vi "Build Do.vi"(4 "BuildType":T1 items=["simple", "Dialog", "PVUpdate", "Dialog&PV", "Asynch", "AsynchDial", "Ack"], 6 "Wiring Spec":T2, 8 "error in (no error)":errorcluster, 10 "Do VI":refnum<vi>, 11 "CS++Actor in":refnum<class "CS++Actor.lvclass">) -> (0 "error out":errorcluster, 3 "CS++Actor out":refnum<class "CS++Actor.lvclass">)   [LabVIEW 2016, in "CS++Actor.lvlib" / "CS++Actor.lvclass"]
doc: "Creates the Do.vi for the new message."
uses:
  CS++Actor.lvclass
  CSPP_MessageMakerMain/BuildType.ctl
  CS++Actor.lvclass/CS++Actor.ctl
  <vilib>/Utility/traverseref.llb/TRef TravTarget.ctl
  <vilib>/Utility/miscctls.llb/LVPositionTypeDef.ctl
  <vilib>/Utility/Data Type/Type Definitions/Data Type.ctl
  <vilib>/Utility/traverseref.llb/VI Scripting - Traverse.lvlib
  <vilib>/Utility/Data Type/NI_Data Type.lvlib
  CSPP_MessageMakerMain/CS++MessageMakerMain.lvclass
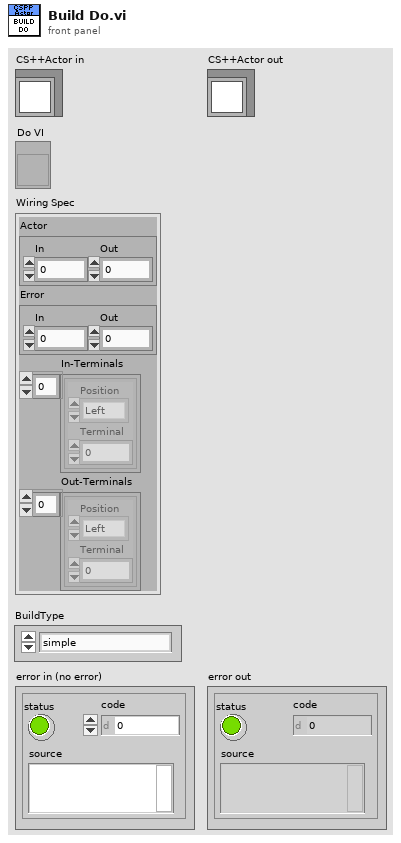
[diagram p1: front panel]
types:
  T1 = typedef "CS++MessageMakerMain.lvlib/CS++MessageMakerMain.lvclass/BuildType.ctl" = u16
  T2 = cluster{"Actor":cluster{"In":i32, "Out":i32}, "Error":cluster{"In":i32, "Out":i32}, "In-Terminals":cluster{"Position":enum16{"Left", "Top", "Bottom", "Right"}, "Terminal":i32}[], "Out-Terminals":cluster{"Position":enum16{"Left", "Top", "Bottom", "Right"}, "Terminal":i32}[]}
  T3 = enum16{"Replace Class Controls/Constants", "Prepare SubVI", "Wire Method Inputs", "Replace Msg Ctrl if necessary", "Create DynamicDispatch Control", "Create PseudoTypedef", "Connect Pre (Un)Bundler", "Replace PV VIs", "RedoWiring", "Connect MethodOut to Bundler", "Delete AsynchAndNoPara", "DeleteBoolDIMConversion"}
  T4 = typedef "TRef TravTarget.ctl" = enum16{"FP", "BD", "Other"}
  T5 = enum16{"Invalid Wire Rule", "Required", "Recommended", "Optional", "Dynamic Dispatch"}
  T6 = typedef "LVPositionTypeDef.ctl" = cluster{"Left":i32, "Top":i32}
  T7 = typedef "NI_Data Type.lvlib/Data Type.ctl" = enum8{"Invalid Type", "Void", "I8", "I16", "I32", "I64", "U8", "U16", "U32", "U64", "Single Float", "Double Float", "Extended Float", "Single Complex", "Double Complex", "Extended Complex", "Enum U8", "Enum U16", "Enum U32", "Enum U64", "Single Float With Unit", "Double Float With Unit", "Extended Float With Unit", "Single Complex with Unit", "Double Complex with Unit", "Extended Complex with Unit", "Boolean", "String", "Path", "Picture", "Tag", "Array", "Cluster", "Variant", "LV Variant", "Waveform", "Timestamp", "Digital Waveform", "Digital Data", "ExpressData", "Refnum", "External Data", "VI", "Poly VI", "LabVIEW Class Instance", "Fixed Point"}
  T8 = cluster{"Position":enum16{"Left", "Top", "Bottom", "Right"}, "Terminal":i32}[]
  T9 = cluster{"Position":enum16{"Left", "Top", "Bottom", "Right"}, "Terminal":i32}
  T10 = enum16{"Invalid Wire Rule", "Required", "Recommended", "Optional", "Dynamic Dispatch"}[]
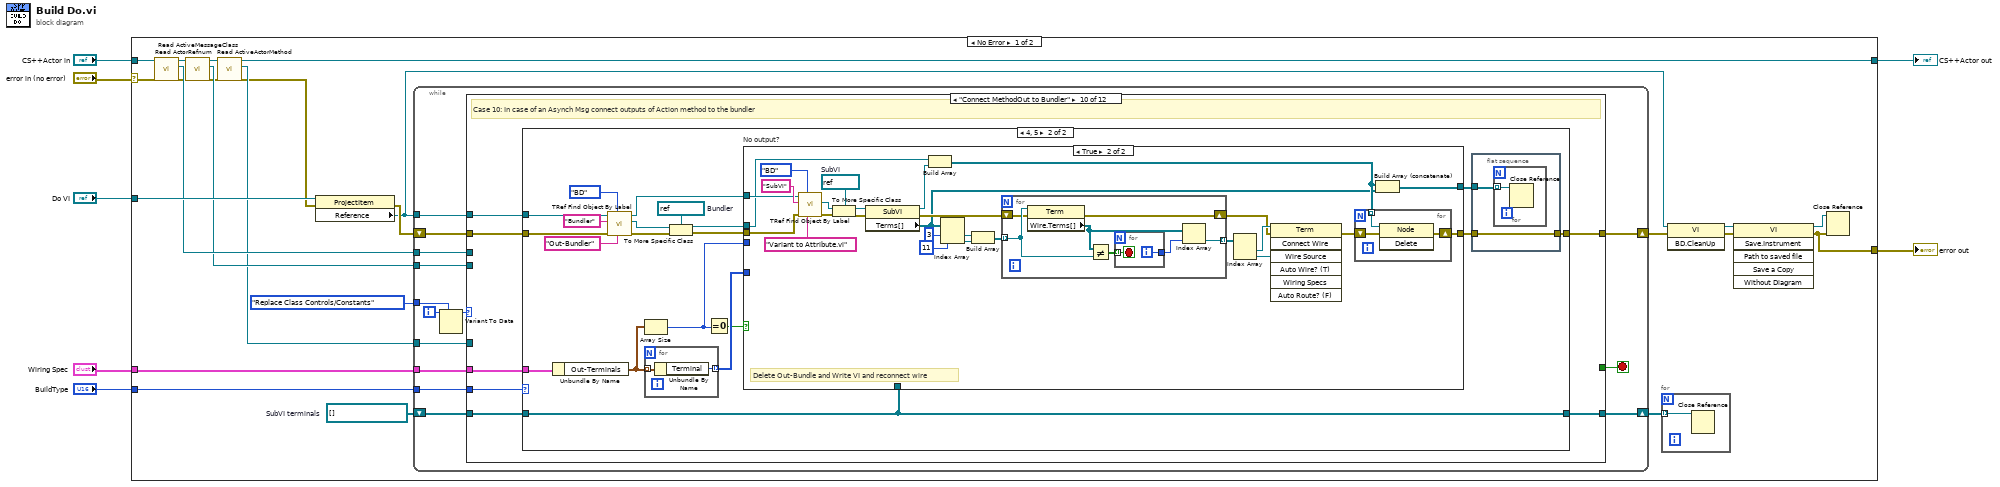
[diagram p0: block diagram]
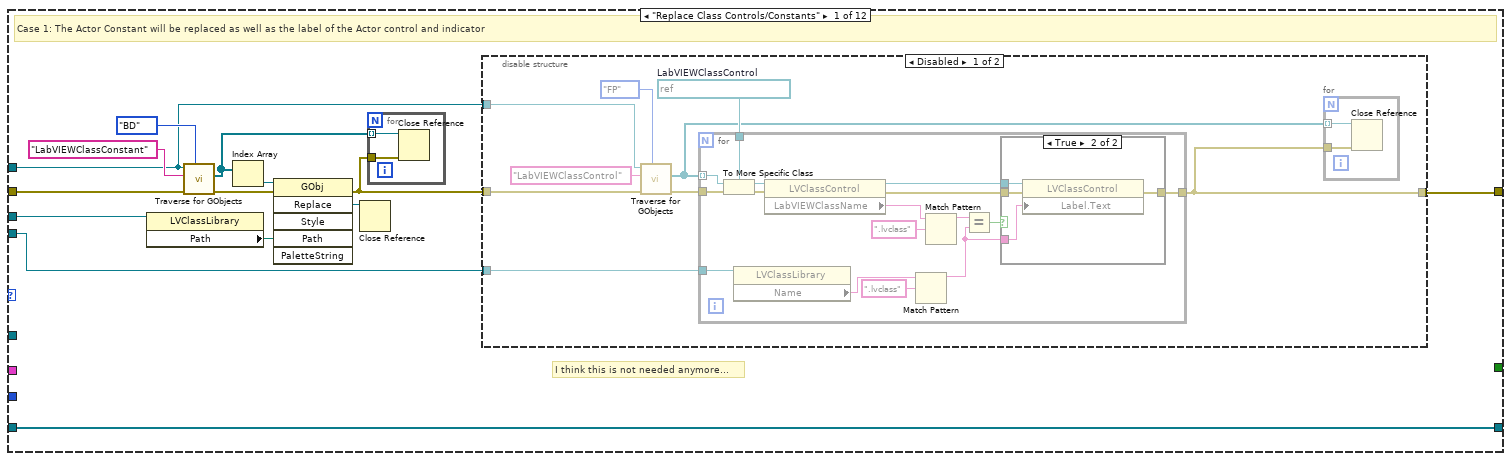
[diagram p2: hidden frame]
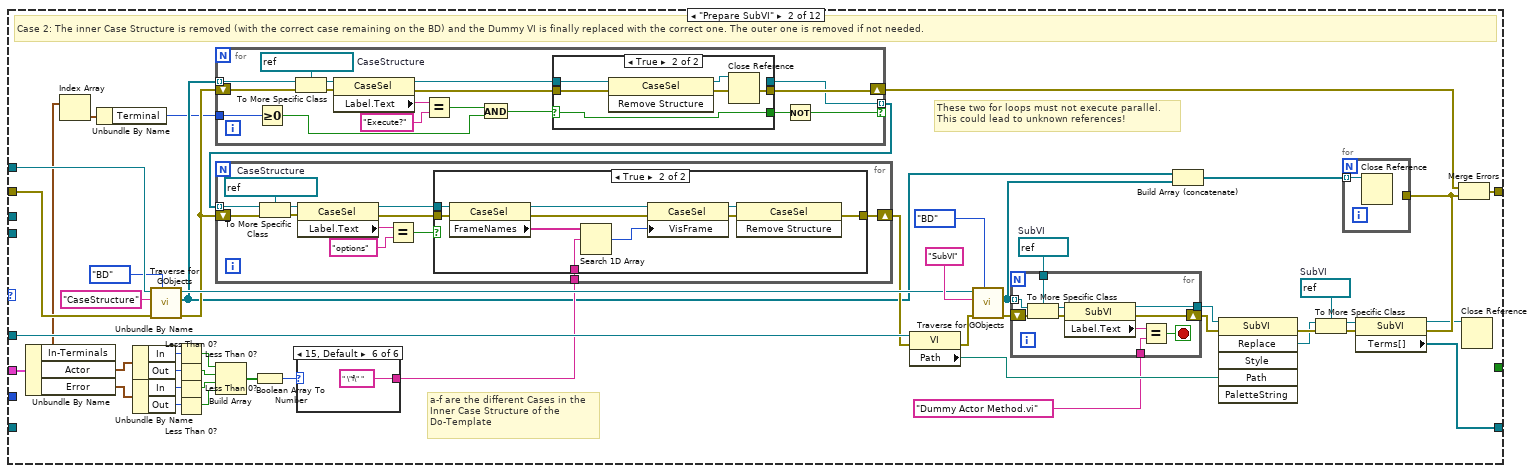
[diagram p5: hidden frame]
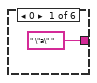
[diagram p8: hidden frame]
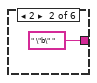
[diagram p9: hidden frame]
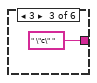
[diagram p10: hidden frame]
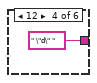
[diagram p11: hidden frame]
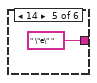
[diagram p12: hidden frame]
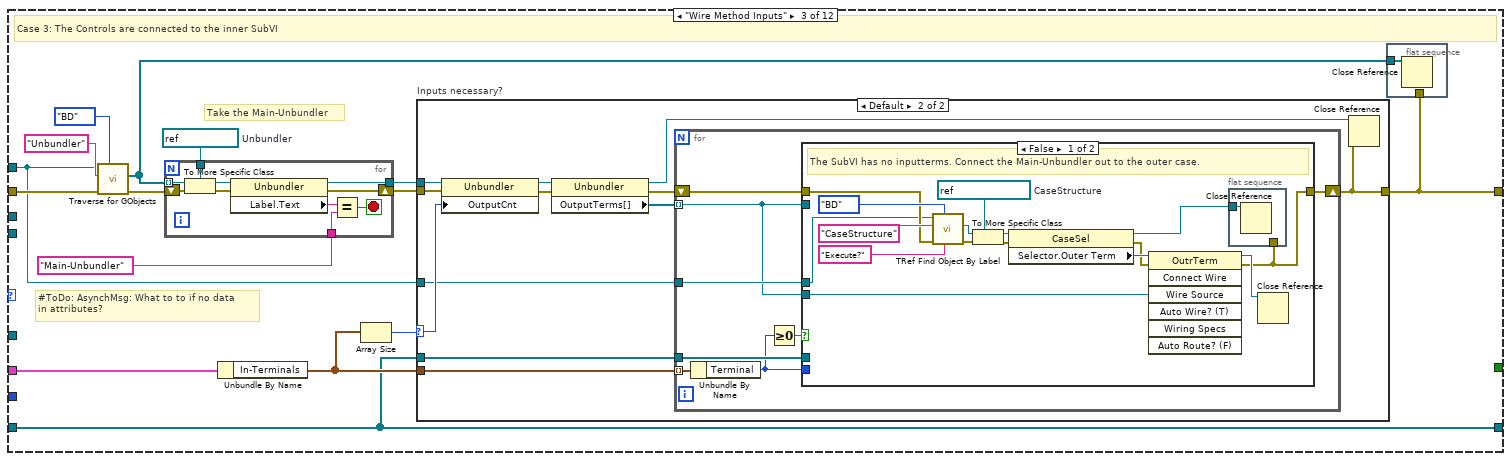
[diagram p13: hidden frame]
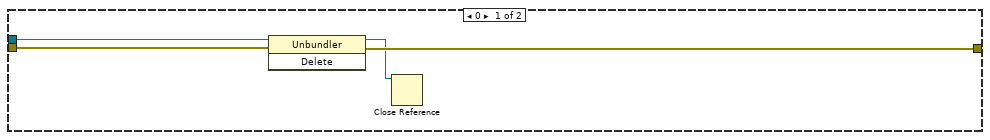
[diagram p14: hidden frame]
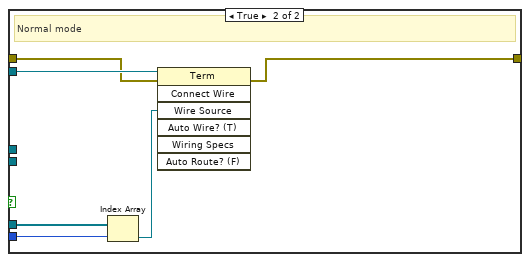
[diagram p15: hidden frame]
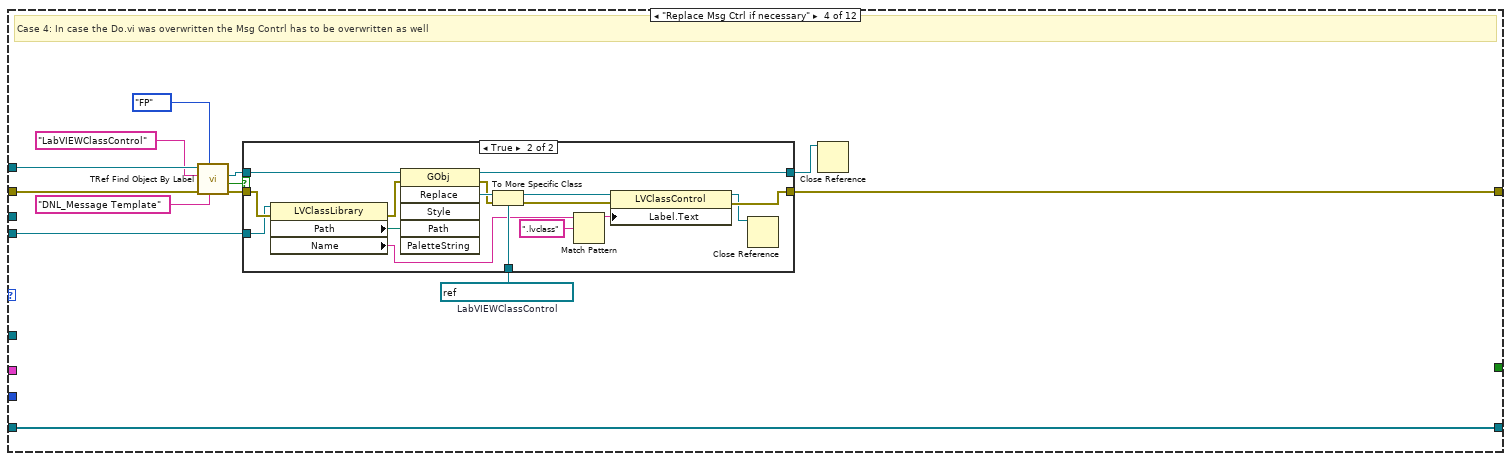
[diagram p16: hidden frame]
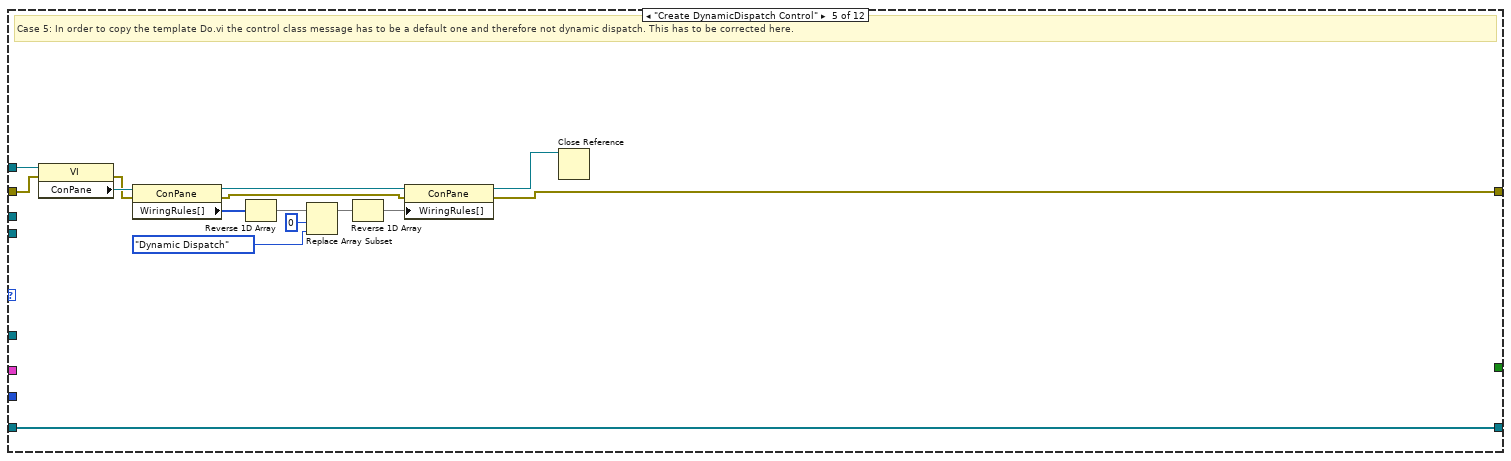
[diagram p18: hidden frame]
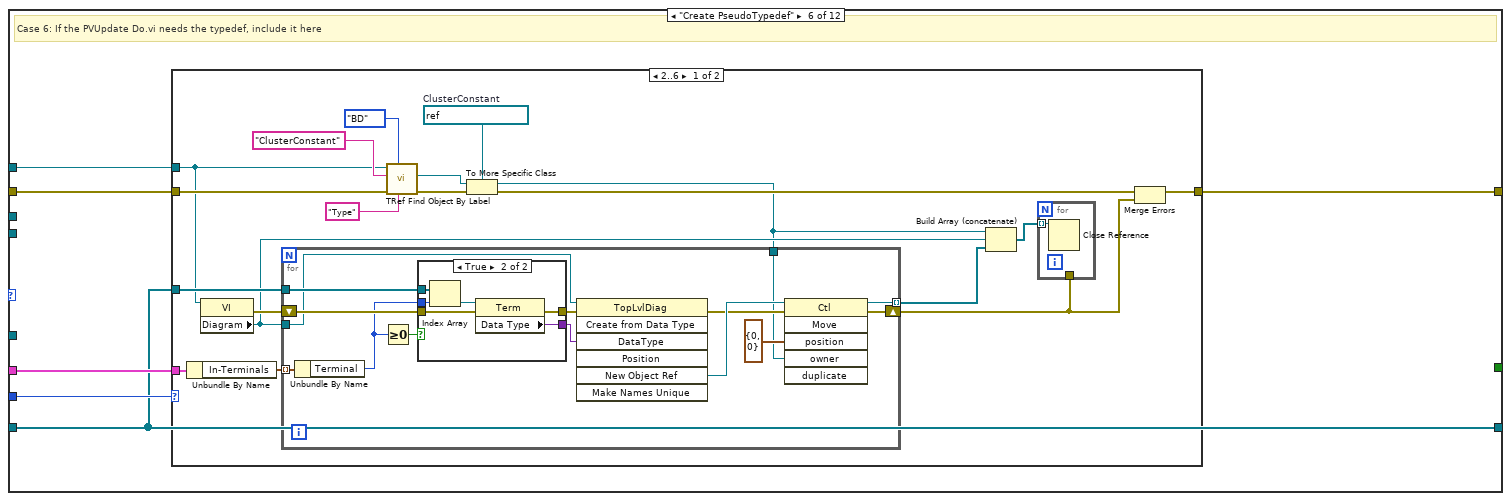
[diagram p19: hidden frame]
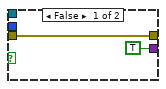
[diagram p20: hidden frame]
diagram:
  n1 = case shown="No Error" "error in (no error)" {
    selector: "error in (no error)" -> [w14 w1120]
    tunnel: "Do VI" -> [w31 _]
    tunnel: "Wiring Spec" -> [w29 _]
    tunnel: [w10 w1120] -> w5
    tunnel: "CS++Actor in" -> [w24 w1121]
    tunnel: [w15 w1121] -> w3
    tunnel: "BuildType" -> [w9 _]
    frame No Error {
      w8 = refnum<vi>[] []  # SubVI terminals
      n2 = call "Read ActorRefnum.vi"("error in (no error)"=w14, "CS++Actor in"=w24) -> ("error out"=w21:errorcluster, "ActorRefnum"=w23:refnum<vi>, "CS++Actor out"=w22:refnum<class "CS++Actor.lvclass">)  [unwired: 7 in]
      n3 = call "Read ActiveMessageClass.vi"("error in (no error)"=w21, "CS++Actor in"=w22) -> ("error out"=w18:errorcluster, "ActiveMessageClass"=w20:refnum<vi>, "CS++Actor out"=w19:refnum<class "CS++Actor.lvclass">)  [unwired: 7 in]
      n4 = call "Read ActiveActorMethod.vi"("error in (no error)"=w18, "CS++Actor in"=w19) -> ("error out"=w16:errorcluster, "ActiveActorMethod"=w17:refnum<vi>, "CS++Actor out"=w15:refnum<class "CS++Actor.lvclass">)  [unwired: 7 in]
      n5 = property class="ProjectItem"(reference=w31, error in=w16) -> (error out=w30:errorcluster, "Reference"=w25:refnum<vi>)  [unwired: 1 out]
      n6 = while {
        tunnel: w25 -> [w46]
        tunnel: w29 -> [w44]
        shift-right: [w43] -> w28
        shift-left: w30 -> [w45]
        tunnel: T3."Replace Class Controls/Constants" -> [w41]
        tunnel: w23 -> [w39]
        tunnel: w17 -> [w38]
        shift-right: [w36] -> w26
        shift-left: w8 -> [w35]
        tunnel: w20 -> [w34]
        tunnel: w9 -> [w33]
        i -> [w42]
        stop <- w37 stop-if-true
        n7 = Variant To Data(type=w41, Variant=w42) -> (data=w40:T3)  [unwired: 1 in, 1 out]
        n8 = case shown="\"Connect MethodOut to Bundler\"" w40 {
          tunnel: w46 -> [w49 w143 w210 w292 w325 w330 w380 w440 w588 w739 w854 w937]
          tunnel: w45 -> [w54 w142 w218 w293 w326 w333 w379 w438 w589 w738 w855 w938]
          tunnel: w44 -> [_ w141 w221 _ _ w329 _ _ _ w737 w853 _]
          tunnel: [w47 w101 w212 w285 w313 w332 w378 w439 w590 w736 w856 w939] -> w43
          tunnel: w39 -> [w55 _ _ _ _ _ _ w437 _ _ _ _]
          tunnel: w38 -> [_ w140 _ _ _ _ _ _ _ _ _ _]
          tunnel: [_ _ _ _ _ _ _ _ _ _ _ TRUE] -> w37
          tunnel: [w51 w139 w209 w294 w327 w328 w381 w441 w592 w742 w858 w941] -> w36
          tunnel: w35 -> [w51 _ w209 w294 w327 w328 w381 w441 w592 w741 w858 w941]
          tunnel: w34 -> [w48 _ _ w284 _ _ _ _ _ _ _ _]
          tunnel: w33 -> [_ _ _ _ _ w331 w377 w436 w591 w740 w857 w940]
          frame "Replace Class Controls/Constants" {
            # "I think this is not needed anymore..."
            # "Case 1: The Actor Constant will be replaced as well as the label of the Actor control and indicator"
            n9 = property class="LVClassLibrary"(reference=w55) -> ("Path"=w58:path)  [unwired: 1 in, 2 out]
            n10 = call <vilib>:"Traverse for GObjects.vi"("Traverse Target"=TRef_TravTarget."BD", "error in (no error)"=w54, "Class Name"="LabVIEWClassConstant", "VI Refnum"=w49) -> ("error out"=w59:errorcluster, "References"=w53:refnum<vi>[])  [unwired: 4 in, 2 out]
            n11 = Index Array(array=w53) -> (element=w57:refnum<vi>)  [unwired: 1 in]
            n12 = invoke class="GObj" method="Replace"(reference=w57, error in=w59, "Path"=w58) -> (error out=w50:errorcluster, "Replace"=w52:refnum<vi>)  [unwired: 3 in, 4 out]
            n13 = Close Reference(reference=w52) -> ()  [unwired: 1 in, 1 out]
            n14 = for {
              tunnel: w53 -> [w95] mode=indexing
              tunnel: w50 -> [w94]
              n15 = Close Reference(reference=w95, error in (no error)=w94) -> ()  [unwired: 1 out]
            }
            n16 = disable-structure shown="Disabled" {
              disable-tunnel: w50 -> [w69 w93]
              disable-tunnel: w49 -> [w68 _]
              disable-tunnel: w48 -> [w63 _]
              disable-tunnel: [w61 w93] -> w47
              frame Disabled {
                w66 = refnum<vi> refnum  # LabVIEWClassControl
                n17 = call <vilib>:"Traverse for GObjects.vi"("Traverse Target"=TRef_TravTarget."FP", "error in (no error)"=w69, "Class Name"="LabVIEWClassControl", "VI Refnum"=w68) -> ("error out"=w64:errorcluster, "References"=w62:refnum<vi>[])  [unwired: 4 in, 2 out]
                n18 = for {
                  tunnel: w66 -> [w87]
                  tunnel: w64 -> [w86]
                  tunnel: w62 -> [w85] mode=indexing
                  tunnel: w63 -> [w80]
                  tunnel: [w82] -> w61
                  n19 = To More Specific Class(target class=w87, reference=w85, error in=w86) -> (specific class reference=w81:refnum<vi>, error out=w83:errorcluster)
                  n20 = property class="LVClassLibrary"(reference=w80) -> ("Name"=w78:string)  [unwired: 1 in, 2 out]
                  n21 = property class="LVClassControl"(reference=w81, error in=w83) -> (reference out=w84:refnum<vi>, error out=w72:errorcluster, "LabVIEWClassName"=w74:string)
                  n22 = Match Pattern(string=w78, regular expression=".lvclass") -> (before substring=w77:string)  [unwired: 1 in, 3 out]
                  n23 = Match Pattern(string=w74, regular expression=".lvclass") -> (before substring=w73:string)  [unwired: 1 in, 3 out]
                  n24 = Equal?(x=w73, y=w77) -> (x = y?=w79:bool)
                  n25 = case shown="True" w79 {
                    tunnel: w84 -> [_ w92]
                    tunnel: [w88 w89] -> w82
                    tunnel: w77 -> [_ w91]
                    tunnel: w72 -> [w88 w90]
                    frame False {
                    }
                    frame True {
                      n26 = property class="LVClassControl"(reference=w92, error in=w90, "Label.Text"=w91) -> (error out=w89:errorcluster)  [unwired: 1 out]
                    }
                  }
                }
                n27 = for {
                  tunnel: w62 -> [w71] mode=indexing
                  tunnel: w61 -> [w70]
                  n28 = Close Reference(reference=w71, error in (no error)=w70) -> ()  [unwired: 1 out]
                }
              }
              frame Enabled {
              }
            }
          }
          frame "Prepare SubVI" {
            w107 = refnum<vi> refnum  # SubVI
            w116 = refnum<vi> refnum  # SubVI
            # "These two for loops must not execute parallel.\nThis could lead to unknown references!"
            # "a-f are the different Cases in the\nInner Case Structure of the \nDo-Template"
            # "Case 2: The inner Case Structure is removed (with the correct case remaining on the BD) and the Dummy VI is finally replaced with the correct one. The outer one is removed if not needed."
            n29 = Unbundle By Name(w141) -> ("In-Terminals"=w99:T8, "Actor"=w136:cluster{"In":i32, "Out":i32}, "Error"=w135:cluster{"In":i32, "Out":i32})
            n30 = Index Array(array=w99) -> (element=w98:T9)  [unwired: 1 in]
            n31 = Unbundle By Name(w98) -> ("Terminal"=w97:i32)
            n32 = Unbundle By Name(w136) -> ("In"=w134:i32, "Out"=w133:i32)
            n33 = Unbundle By Name(w135) -> ("In"=w132:i32, "Out"=w131:i32)
            n34 = call <vilib>:"Traverse for GObjects.vi"("Traverse Target"=TRef_TravTarget."BD", "error in (no error)"=w142, "Class Name"="CaseStructure", "VI Refnum"=w143) -> ("error out"=w105:errorcluster, "References"=w102:refnum<vi>[], "dup VI Refnum"=w124:refnum<vi>)  [unwired: 4 in, 1 out]
            n35 = Less Than 0?(x=w134) -> (x < 0?=w130:bool)
            n36 = Less Than 0?(x=w133) -> (x < 0?=w129:bool)
            n37 = Less Than 0?(x=w132) -> (x < 0?=w128:bool)
            n38 = Less Than 0?(x=w131) -> (x < 0?=w127:bool)
            n39 = for {
              tunnel: w102 -> [w155] mode=indexing
              shift-right: [w152] -> w100
              shift-left: w105 -> [w156]
              tunnel: w97 -> [w151]
              tunnel: [w146] -> w96 mode=indexing if=w144
              w160 = refnum<vi> refnum  # CaseStructure
              n40 = Greater Or Equal To 0?(x=w151) -> (x >= 0?=w147:bool)
              n41 = To More Specific Class(target class=w160, reference=w155, error in=w156) -> (specific class reference=w159:refnum<vi>, error out=w158:errorcluster)
              n42 = property class="CaseSel"(reference=w159, error in=w158) -> (reference out=w154:refnum<vi>, error out=w153:errorcluster, "Label.Text"=w150:string)
              n43 = Equal?(x=w150, y="Execute?") -> (x = y?=w149:bool)
              n44 = And(x=w149, y=w147) -> (x .and. y?=w148:bool)
              n45 = case shown="True" w148 {
                selector: w148 -> [w161 w165]
                tunnel: w154 -> [w162 w168]
                tunnel: w153 -> [w163 w167]
                tunnel: [w163 w166] -> w152
                tunnel: [w162 _] -> w146
                tunnel: [w161 w165] -> w145
                frame False {
                }
                frame True {
                  n46 = invoke class="CaseSel" method="Remove Structure"(reference=w168, error in=w167) -> (reference out=w164:refnum<vi>, error out=w166:errorcluster)  [unwired: 1 in, 1 out]
                  n47 = Close Reference(reference=w164) -> ()  [unwired: 1 in, 1 out]
                }
              }
              n48 = Not(x=w145) -> (.not. x?=w144:bool)
            }
            n49 = Build Array(w130, w129, w128, w127) -> (w126:bool[])
            n50 = Boolean Array To Number(Boolean array=w126) -> (number=w125:u32)
            n51 = case shown="15, Default" w125 {
              tunnel: [" \"a\" " " \"b\" " " \"c\" " " \"d\" " " \"e\" " " \"f\" "] -> w121
              frame 0 {
              }
              frame 2 {
              }
              frame 3 {
              }
              frame 12 {
              }
              frame 14 {
              }
              frame 15, Default {
              }
            }
            n52 = for {
              tunnel: w96 -> [w181] mode=indexing
              tunnel: w121 -> [w172]
              shift-right: [w170] -> w119
              shift-left: w105 -> [w171]
              w180 = refnum<vi> refnum  # CaseStructure
              n53 = To More Specific Class(target class=w180, reference=w181, error in=w171) -> (specific class reference=w179:refnum<vi>, error out=w178:errorcluster)
              n54 = property class="CaseSel"(reference=w179, error in=w178) -> (reference out=w174:refnum<vi>, error out=w173:errorcluster, "Label.Text"=w177:string)
              n55 = Equal?(x=w177, y="options") -> (x = y?=w175:bool)
              n56 = case shown="True" w175 {
                tunnel: w174 -> [_ w190]
                tunnel: w173 -> [w182 w188]
                tunnel: w172 -> [_ w184]
                tunnel: [w182 w183] -> w170
                frame False {
                }
                frame True {
                  n57 = property class="CaseSel"(reference=w190, error in=w188) -> (reference out=w189:refnum<vi>, error out=w187:errorcluster, "FrameNames"=w186:string[])
                  n58 = Search 1D Array(1D array=w186, element=w184) -> (index of element=w185:i32)  [unwired: 1 in]
                  n59 = property class="CaseSel"(reference=w189, error in=w187, "VisFrame"=w185) -> (reference out=w192:refnum<vi>, error out=w191:errorcluster)
                  n60 = invoke class="CaseSel" method="Remove Structure"(reference=w192, error in=w191) -> (error out=w183:errorcluster)  [unwired: 1 in, 2 out]
                }
              }
            }
            n61 = property class="VI"(reference=w140, error in=w119) -> (error out=w118:errorcluster, "Path"=w117:path)  [unwired: 1 out]
            n62 = call <vilib>:"Traverse for GObjects.vi"("Traverse Target"=TRef_TravTarget."BD", "error in (no error)"=w118, "Class Name"="SubVI", "VI Refnum"=w124) -> ("error out"=w120:errorcluster, "References"=w104:refnum<vi>[])  [unwired: 4 in, 2 out]
            n63 = for {
              tunnel: w104 -> [w207] mode=indexing
              tunnel: w116 -> [w206]
              tunnel: [w201] -> w115
              shift-right: [w200] -> w114
              shift-left: w120 -> [w208]
              tunnel: "Dummy Actor Method.vi" ("Class Name") -> [w199]
              stop <- w202 stop-if-true
              n64 = To More Specific Class(target class=w206, reference=w207, error in=w208) -> (specific class reference=w205:refnum<vi>, error out=w204:errorcluster)
              n65 = property class="SubVI"(reference=w205, error in=w204) -> (reference out=w201:refnum<vi>, error out=w200:errorcluster, "Label.Text"=w203:string)
              n66 = Equal?(x=w203, y=w199) -> (x = y?=w202:bool)
            }
            n67 = Build Array (concatenate)(w102, w104) -> (w103:refnum<vi>[])
            n68 = invoke class="SubVI" method="Replace"(reference=w115, error in=w114, "Path"=w117) -> (error out=w110:errorcluster, "Replace"=w109:refnum<vi>)  [unwired: 3 in, 4 out]
            n69 = To More Specific Class(target class=w107, reference=w109, error in=w110) -> (specific class reference=w108:refnum<vi>, error out=w111:errorcluster)
            n70 = property class="SubVI"(reference=w108, error in=w111) -> (reference out=w106:refnum<vi>, error out=w112:errorcluster, "Terms[]"=w139:refnum<vi>[])
            n71 = for {
              tunnel: w103 -> [w169] mode=indexing
              tunnel: w112 -> [_]
              n72 = Close Reference(reference=w169) -> ()  [unwired: 1 in, 1 out]
            }
            n73 = Merge Errors(w100, w112) -> (w101:errorcluster)
            n74 = Close Reference(reference=w106) -> ()  [unwired: 1 in, 1 out]
          }
          frame "Wire Method Inputs" {
            w216 = refnum<vi> refnum  # Unbundler
            # "#ToDo: AsynchMsg: What to to if no data\nin attributes?"
            # "Take the Main-Unbundler"
            # "Case 3: The Controls are connected to the inner SubVI"
            n75 = call <vilib>:"Traverse for GObjects.vi"("Traverse Target"=TRef_TravTarget."BD", "error in (no error)"=w218, "Class Name"="Unbundler", "VI Refnum"=w210) -> ("error out"=w217:errorcluster, "References"=w211:refnum<vi>[])  [unwired: 4 in, 2 out]
            n76 = for {
              tunnel: w211 -> [w233] mode=indexing
              tunnel: w216 -> [w230]
              tunnel: "Main-Unbundler" ("Class Name") -> [w228]
              shift-right: [w227] -> w213
              shift-left: w217 -> [w234]
              tunnel: [w226] -> w214
              stop <- w225 stop-if-true
              n77 = To More Specific Class(target class=w230, reference=w233, error in=w234) -> (specific class reference=w232:refnum<vi>, error out=w231:errorcluster)
              n78 = property class="Unbundler"(reference=w232, error in=w231) -> (reference out=w226:refnum<vi>, error out=w227:errorcluster, "Label.Text"=w229:string)
              n79 = Equal?(x=w229, y=w228) -> (x = y?=w225:bool)
            }
            n80 = Unbundle By Name(w221) -> ("In-Terminals"=w219:T8)
            n81 = Array Size(array=w219) -> (size(s)=w220:i32)
            n82 = case "Inputs necessary?" shown="Default" w220 {
              selector: w220 -> [_ w245]
              tunnel: w214 -> [w238 w243]
              tunnel: w209 -> [_ w248]
              tunnel: w213 -> [w237 w240]
              tunnel: [w236 w241] -> w212
              tunnel: w219 -> [_ w250]
              tunnel: w210 -> [_ w239]
              frame 0 {
                n83 = invoke class="Unbundler" method="Delete"(reference=w238, error in=w237) -> (reference out=w235:refnum<vi>, error out=w236:errorcluster)  [unwired: 1 in, 1 out]
                n84 = Close Reference(reference=w235) -> ()  [unwired: 1 in, 1 out]
              }
              frame Default {
                n85 = property class="Unbundler"(reference=w243, error in=w240, "OutputCnt"=w245) -> (reference out=w246:refnum<vi>, error out=w244:errorcluster)
                n86 = property class="Unbundler"(reference=w246, error in=w244) -> (reference out=w242:refnum<vi>, error out=w247:errorcluster, "OutputTerms[]"=w249:refnum<vi>[])
                n87 = for {
                  tunnel: w250 -> [w255] mode=indexing
                  tunnel: w249 -> [w251] mode=indexing
                  tunnel: w248 -> [w258]
                  shift-right: [w256] -> w241
                  shift-left: w247 -> [w257]
                  tunnel: w239 -> [w252]
                  n88 = Unbundle By Name(w255) -> ("Terminal"=w254:i32)
                  n89 = Greater Or Equal To 0?(x=w254) -> (x >= 0?=w253:bool)
                  n90 = case shown="False" w253 {
                    tunnel: w251 -> [_ w281]
                    tunnel: w258 -> [_ w280]
                    tunnel: w257 -> [w265 w278]
                    tunnel: [w260 w277] -> w256
                    tunnel: w254 -> [_ w276]
                    tunnel: w252 -> [w264 _]
                    tunnel: w251 -> [w263 _]
                    frame False {
                      w270 = refnum<vi> refnum  # CaseStructure
                      # "The SubVI has no inputterms. Connect the Main-Unbundler out to the outer case."
                      n91 = call <vilib>:"TRef Find Object By Label.vi"("Label"="Execute?", "Traverse Target"=TRef_TravTarget."BD", "error in (no error)"=w265, "Class Name"="CaseStructure", "VI Ref"=w264) -> ("error out"=w271:errorcluster, "Found Obj Ref"=w272:refnum<vi>)  [unwired: 3 in, 2 out]
                      n92 = To More Specific Class(target class=w270, reference=w272, error in=w271) -> (specific class reference=w269:refnum<vi>, error out=w268:errorcluster)
                      n93 = property class="CaseSel"(reference=w269, error in=w268) -> (reference out=w259:refnum<vi>, error out=w262:errorcluster, "Selector.Outer Term"=w267:refnum<vi>)
                      n94 = invoke class="OutrTerm" method="Connect Wire"(reference=w267, error in=w262, "Wire Source"=w263) -> (reference out=w261:refnum<vi>, error out=w260:errorcluster)  [unwired: 4 in, 5 out]
                      n95 = flat-sequence {
                        tunnel: w260 -> [_]
                        tunnel: w259 -> [w275]
                        frame #0 {
                          n96 = Close Reference(reference=w275) -> ()  [unwired: 1 in, 1 out]
                        }
                      }
                      n97 = Close Reference(reference=w261) -> ()  [unwired: 1 in, 1 out]
                    }
                    frame True {
                      # "Normal mode"
                      n98 = Index Array(array=w280, index=w276) -> (element=w279:refnum<vi>)
                      n99 = invoke class="Term" method="Connect Wire"(reference=w281, error in=w278, "Wire Source"=w279) -> (error out=w277:errorcluster)  [unwired: 4 in, 6 out]
                    }
                  }
                }
                n100 = Close Reference(reference=w242, error in (no error)=w241) -> ()  [unwired: 1 out]
              }
            }
            n101 = flat-sequence {
              tunnel: w212 -> [_]
              tunnel: w211 -> [w224]
              frame #0 {
                n102 = Close Reference(reference=w224) -> ()  [unwired: 1 in, 1 out]
              }
            }
          }
          frame "Replace Msg Ctrl if necessary" {
            w282 = refnum<vi> refnum  # LabVIEWClassControl
            # "Case 4: In case the Do.vi was overwritten the Msg Contrl has to be overwritten as well"
            n103 = call <vilib>:"TRef Find Object By Label.vi"("Label"="DNL_Message Template", "Traverse Target"=TRef_TravTarget."FP", "error in (no error)"=w293, "Class Name"="LabVIEWClassControl", "VI Ref"=w292) -> ("error out"=w288:errorcluster, "Found?"=w289:bool, "Found Obj Ref"=w287:refnum<vi>)  [unwired: 3 in, 1 out]
            n104 = case shown="True" w289 {
              tunnel: w288 -> [w295 w309]
              tunnel: w287 -> [w296 w311]
              tunnel: [w296 w310] -> w286
              tunnel: [w295 w301] -> w285
              tunnel: w284 -> [_ w307]
              tunnel: w282 -> [_ w305]
              frame False {
              }
              frame True {
                n105 = property class="LVClassLibrary"(reference=w307, error in=w309) -> (error out=w308:errorcluster, "Path"=w312:path, "Name"=w299:string)  [unwired: 1 out]
                n106 = invoke class="GObj" method="Replace"(reference=w311, error in=w308, "Path"=w312) -> (reference out=w310:refnum<vi>, error out=w302:errorcluster, "Replace"=w306:refnum<vi>)  [unwired: 3 in, 3 out]
                n107 = To More Specific Class(target class=w305, reference=w306, error in=w302) -> (specific class reference=w304:refnum<vi>, error out=w303:errorcluster)
                n108 = Match Pattern(string=w299, regular expression=".lvclass") -> (before substring=w298:string)  [unwired: 1 in, 3 out]
                n109 = property class="LVClassControl"(reference=w304, error in=w303, "Label.Text"=w298) -> (reference out=w300:refnum<vi>, error out=w301:errorcluster)
                n110 = Close Reference(reference=w300) -> ()  [unwired: 1 in, 1 out]
              }
            }
            n111 = Close Reference(reference=w286) -> ()  [unwired: 1 in, 1 out]
          }
          frame "Create DynamicDispatch Control" {
            # "Case 5: In order to copy the template Do.vi the control class message has to be a default one and therefore not dynamic dispatch. This has to be corrected here."
            n112 = property class="VI"(reference=w325, error in=w326) -> (error out=w323:errorcluster, "ConPane"=w324:refnum<vi>)  [unwired: 1 out]
            n113 = property class="ConPane"(reference=w324, error in=w323) -> (reference out=w315:refnum<vi>, error out=w316:errorcluster, "WiringRules[]"=w322:T10)
            n114 = Reverse 1D Array(array=w322) -> (reversed array=w321:T10)
            n115 = Replace Array Subset(array=w321, new element=T5."Dynamic Dispatch" ("new element/subarray"), index=0) -> (w320:T10)
            n116 = Reverse 1D Array(array=w320) -> (reversed array=w319:T10)
            n117 = property class="ConPane"(reference=w315, error in=w316, "WiringRules[]"=w319) -> (reference out=w314:refnum<vi>, error out=w313:errorcluster)
            n118 = Close Reference(reference=w314) -> ()  [unwired: 1 in, 1 out]
          }
          frame "Create PseudoTypedef" {
            # "Case 6: If the PVUpdate Do.vi needs the typedef, include it here"
            n119 = case shown="2..6" w331 {
              tunnel: w333 -> [w350 w376]
              tunnel: [w341 w376] -> w332
              tunnel: w330 -> [w344 _]
              tunnel: w329 -> [w348 _]
              tunnel: w328 -> [w345 _]
              frame 2..6 {
                w346 = refnum<vi> refnum  # ClusterConstant
                n120 = Unbundle By Name(w348) -> ("In-Terminals"=w347:T8)
                n121 = property class="VI"(reference=w344) -> (error out=w343:errorcluster, "Diagram"=w339:refnum<vi>)  [unwired: 1 in, 1 out]
                n122 = call <vilib>:"TRef Find Object By Label.vi"("Label"="Type", "Traverse Target"=TRef_TravTarget."BD", "error in (no error)"=w350, "Class Name"="ClusterConstant", "VI Ref"=w344) -> ("error out"=w336:errorcluster, "Found Obj Ref"=w335:refnum<vi>)  [unwired: 3 in, 2 out]
                n123 = To More Specific Class(target class=w346, reference=w335, error in=w336) -> (specific class reference=w334:refnum<vi>, error out=w342:errorcluster)
                n124 = for {
                  tunnel: w347 -> [w367] mode=indexing
                  tunnel: w345 -> [w366]
                  shift-right: [w359] -> w340
                  shift-left: w343 -> [w363]
                  tunnel: w339 -> [w362]
                  tunnel: w334 -> [w357]
                  tunnel: [w356] -> w338 mode=indexing
                  n125 = Unbundle By Name(w367) -> ("Terminal"=w354:i32)
                  n126 = Greater Or Equal To 0?(x=w354) -> (x >= 0?=w355:bool)
                  n127 = case shown="True" w355 {
                    tunnel: w366 -> [_ w375]
                    tunnel: w354 -> [_ w374]
                    tunnel: [w369 w372] -> w365
                    tunnel: [TRUE w371] -> w364
                    tunnel: w363 -> [w369 w370]
                    frame False {
                    }
                    frame True {
                      n128 = Index Array(array=w375, index=w374) -> (element=w373:refnum<vi>)
                      n129 = property class="Term"(reference=w373, error in=w370) -> (error out=w372:errorcluster, "Data Type"=w371:variant)  [unwired: 1 out]
                    }
                  }
                  n130 = invoke class="TopLvlDiag" method="Create from Data Type"(reference=w362, error in=w365, "DataType"=w364) -> (error out=w360:errorcluster, "New Object Ref"=w361:refnum<vi>)  [unwired: 4 in, 5 out]
                  n131 = invoke class="Ctl" method="Move"(reference=w361, error in=w360, "position"=T6 {"Left"=0, "Top"=0}, "owner"=w357) -> (reference out=w356:refnum<vi>, error out=w359:errorcluster)  [unwired: 2 in, 4 out]
                }
                n132 = Build Array (concatenate)(w334, w339, w338) -> (w337:refnum<vi>[])
                n133 = for {
                  tunnel: w340 -> [_]
                  tunnel: w337 -> [w353] mode=indexing
                  n134 = Close Reference(reference=w353) -> ()  [unwired: 1 in, 1 out]
                }
                n135 = Merge Errors(w342, w340) -> (w341:errorcluster)
              }
              frame Default {
              }
            }
          }
          frame "Connect Pre (Un)Bundler" {
            # "Case 7: For the PVUpdate Do.vi this case connects the pre (un)bundler"
            n136 = case shown="2, 3" w377 {
              tunnel: w380 -> [_ w405]
              tunnel: w379 -> [w382 w404]
              tunnel: [w382 w383] -> w378
              frame Default {
              }
              frame 2, 3 {
                w400 = refnum<vi> refnum  # Bundler
                w407 = refnum<vi> refnum  # Unbundler
                # "Take the Pre-Bundler"
                # "Take the Pre-Unbundler"
                n137 = call <vilib>:"Traverse for GObjects.vi"("Traverse Target"=TRef_TravTarget."BD", "error in (no error)"=w404, "Class Name"="Unbundler", "VI Refnum"=w405) -> ("error out"=w408:errorcluster, "References"=w385:refnum<vi>[], "dup VI Refnum"=w397:refnum<vi>)  [unwired: 4 in, 1 out]
                n138 = for {
                  tunnel: w385 -> [w434] mode=indexing
                  tunnel: w407 -> [w431]
                  tunnel: "Pre-Unbundler" ("Class Name") -> [w429]
                  shift-right: [w428] -> w398
                  shift-left: w408 -> [w435]
                  tunnel: [w427] -> w396
                  stop <- w426 stop-if-true
                  n139 = To More Specific Class(target class=w431, reference=w434, error in=w435) -> (specific class reference=w433:refnum<vi>, error out=w432:errorcluster)
                  n140 = property class="Unbundler"(reference=w433, error in=w432) -> (reference out=w427:refnum<vi>, error out=w428:errorcluster, "Label.Text"=w430:string)
                  n141 = Equal?(x=w430, y=w429) -> (x = y?=w426:bool)
                }
                n142 = call <vilib>:"Traverse for GObjects.vi"("Traverse Target"=TRef_TravTarget."BD", "error in (no error)"=w398, "Class Name"="Bundler", "VI Refnum"=w397) -> ("error out"=w401:errorcluster, "References"=w386:refnum<vi>[])  [unwired: 4 in, 2 out]
                n143 = for {
                  tunnel: w386 -> [w424] mode=indexing
                  tunnel: w400 -> [w421]
                  tunnel: "Pre-Bundler" ("Class Name") -> [w419]
                  shift-right: [w418] -> w394
                  shift-left: w401 -> [w425]
                  tunnel: [w417] -> w395
                  stop <- w416 stop-if-true
                  n144 = To More Specific Class(target class=w421, reference=w424, error in=w425) -> (specific class reference=w423:refnum<vi>, error out=w422:errorcluster)
                  n145 = property class="Bundler"(reference=w423, error in=w422) -> (reference out=w417:refnum<vi>, error out=w418:errorcluster, "Label.Text"=w420:string)
                  n146 = Equal?(x=w420, y=w419) -> (x = y?=w416:bool)
                }
                n147 = property class="Unbundler"(reference=w396, error in=w394) -> (error out=w392:errorcluster, "OutputTerms[]"=w387:refnum<vi>[])  [unwired: 1 out]
                n148 = Array Size(array=w387) -> (size(s)=w393:i32)
                n149 = property class="Bundler"(reference=w395, error in=w392, "InputCnt"=w393) -> (reference out=w391:refnum<vi>, error out=w390:errorcluster)
                n150 = property class="Bundler"(reference=w391, error in=w390) -> (error out=w389:errorcluster, "InputTerms[]"=w388:refnum<vi>[])  [unwired: 1 out]
                n151 = for {
                  tunnel: w387 -> [w414] mode=indexing
                  tunnel: w388 -> [w415] mode=indexing
                  shift-right: [w412] -> w383
                  shift-left: w389 -> [w413]
                  n152 = invoke class="Term" method="Connect Wire"(reference=w415, error in=w413, "Wire Source"=w414) -> (error out=w412:errorcluster)  [unwired: 4 in, 6 out]
                }
                n153 = Build Array (concatenate)(w385, w386, w387, w388) -> (w384:refnum<vi>[])
                n154 = for {
                  tunnel: w384 -> [w411] mode=indexing
                  tunnel: w383 -> [_]
                  n155 = Close Reference(reference=w411) -> ()  [unwired: 1 in, 1 out]
                }
              }
            }
          }
          frame "Replace PV VIs" {
            # "Case 8: Replace the two Dummy VIs to get the data from the PV"
            n156 = case shown="4, 5" w436 {
              tunnel: w440 -> [_ w483 w539 w575]
              tunnel: [w442 w472 w538 w574] -> w439
              tunnel: w438 -> [w442 w471 w537 w573]
              tunnel: w437 -> [_ w470 w536 w572]
              frame Default {
              }
              frame 2, 3 {
                w478 = "SubVI" ("Class Name")
                w479 = TRef_TravTarget."BD" ("Traverse Target")
                n157 = property class="LVClassLibrary"(reference=w470, error in=w471) -> (error out=w468:errorcluster, "Project"=w469:refnum<vi>)  [unwired: 1 out]
                n158 = property class="Project"(reference=w469, error in=w468) -> (reference out=w466:refnum<vi>, error out=w467:errorcluster, "Path"=w444:path)
                n159 = Strip Path(path=w444) -> (stripped path=w443:path)  [unwired: 1 out]
                n160 = Close Reference(reference=w466) -> ()  [unwired: 1 in, 1 out]
                n161 = Build Path(base path=w443, name or relative path="Packages") -> (appended path=w464:path)
                n162 = Build Path(base path=w464, name or relative path="CSPP_Core") -> (appended path=w450:path)
                n163 = Build Path(base path=w450, name or relative path="Actors") -> (appended path=w461:path)
                n164 = Build Path(base path=w461, name or relative path="CS++PVMonitor Messages") -> (appended path=w459:path)
                n165 = call <vilib>:"TRef Find Object By Label.vi"("Label"="Dummy Read PV.vi" ("Class Name"), "Traverse Target"=w479, "error in (no error)"=w467, "Class Name"=w478, "VI Ref"=w483) -> ("error out"=w481:errorcluster, "Found Obj Ref"=w475:refnum<vi>, "dup VI Ref"=w480:refnum<vi>)  [unwired: 3 in, 1 out]
                n166 = Build Path(base path=w459, name or relative path="CS++PVUpdate Msg") -> (appended path=w457:path)
                n167 = Build Path(base path=w457, name or relative path="Read PV.vi") -> (appended path=w455:path)
                n168 = call <vilib>:"TRef Find Object By Label.vi"("Label"="Dummy Read Data.vi" ("Class Name"), "Traverse Target"=w479, "error in (no error)"=w481, "Class Name"=w478, "VI Ref"=w480) -> ("error out"=w476:errorcluster, "Found Obj Ref"=w474:refnum<vi>)  [unwired: 3 in, 2 out]
                n169 = Build Path(base path=w450, name or relative path="Classes") -> (appended path=w453:path)
                n170 = Build Path(base path=w453, name or relative path="CS++ProcessVariables") -> (appended path=w452:path)
                n171 = Build Path(base path=w452, name or relative path="ProcessVariable") -> (appended path=w451:path)
                n172 = Build Path(base path=w451, name or relative path="Read Data.vi") -> (appended path=w445:path)
                n173 = Build Array(w475, w474) -> (w473:refnum<vi>[])
                n174 = Build Array(w455, w445) -> (w454:path[])
                n175 = for {
                  shift-right: [w487] -> w472
                  shift-left: w476 -> [w488]
                  tunnel: w473 -> [w486] mode=indexing
                  tunnel: w454 -> [w484] mode=indexing
                  n176 = invoke class="GObj" method="Replace"(reference=w486, error in=w488, "Path"=w484) -> (reference out=w485:refnum<vi>, error out=w487:errorcluster)  [unwired: 3 in, 4 out]
                  n177 = Close Reference(reference=w485) -> ()  [unwired: 1 in, 1 out]
                }
              }
              frame 4, 5 {
                n178 = property class="LVClassLibrary"(reference=w536, error in=w537) -> (error out=w534:errorcluster, "Project"=w535:refnum<vi>)  [unwired: 1 out]
                n179 = property class="Project"(reference=w535, error in=w534) -> (reference out=w532:refnum<vi>, error out=w533:errorcluster, "Path"=w524:path)
                n180 = Strip Path(path=w524) -> (stripped path=w523:path)  [unwired: 1 out]
                n181 = Build Path(base path=w523, name or relative path="Packages") -> (appended path=w530:path)
                n182 = Close Reference(reference=w532) -> ()  [unwired: 1 in, 1 out]
                n183 = Build Path(base path=w530, name or relative path="CSPP_Core") -> (appended path=w500:path)
                n184 = Build Path(base path=w500, name or relative path="Messages") -> (appended path=w516:path)
                n185 = Build Path(base path=w500, name or relative path="Libraries") -> (appended path=w498:path)
                n186 = Build Path(base path=w516, name or relative path="CS++AsynchReturnMsg") -> (appended path=w512:path)
                n187 = Build Path(base path=w512, name or relative path="Read AcknowledgeMsg.vi") -> (appended path=w511:path)
                n188 = Build Path(base path=w498, name or relative path="Utilities") -> (appended path=w496:path)
                n189 = Build Path(base path=w512, name or relative path="Read CallerParameter.vi") -> (appended path=w508:path)
                n190 = Build Path(base path=w496, name or relative path="Error Cluster from Error Code.vi") -> (appended path=w494:path)
                n191 = Build Path(base path=w512, name or relative path="Write AcknowledgeMsg.vi") -> (appended path=w501:path)
                n192 = VI Library() -> (path=w493:path)
                n193 = for {
                  tunnel: w539 -> [w546]
                  tunnel: string[] ["Dummy Read AckMsg.vi", "Dummy Read Time Stamp.vi", "Dummy Read TimeOut.vi", "Dummy Read CallerParameter.vi", "Dummy Write ReturnParameter.vi", "Dummy Write AckMsg.vi", "Dummy Error Cluster from Error Code.vi", "Dummy Write Expired.vi", "Dummy Write Error.vi"] -> [w540] mode=indexing
                  shift-right: [w542] -> w522
                  shift-left: w533 -> [w543]
                  tunnel: [w541] -> w520 mode=indexing
                  n194 = call <vilib>:"TRef Find Object By Label.vi"("Label"=w540, "Traverse Target"=TRef_TravTarget."BD", "error in (no error)"=w543, "Class Name"="SubVI", "VI Ref"=w546) -> ("error out"=w542:errorcluster, "Found Obj Ref"=w541:refnum<vi>)  [unwired: 3 in, 2 out]
                }
                n195 = Build Path(base path=w493, name or relative path="ActorFramework") -> (appended path=w492:path)
                n196 = Build Path(base path=w492, name or relative path="Message") -> (appended path=w491:path)
                n197 = Build Path(base path=w516, name or relative path="CS++AcknowledgeMsg") -> (appended path=w505:path)
                n198 = Build Path(base path=w505, name or relative path="Read Time Stamp.vi") -> (appended path=w510:path)
                n199 = Build Path(base path=w505, name or relative path="Read TimeOut.vi") -> (appended path=w509:path)
                n200 = Build Path(base path=w491, name or relative path="Variant to Attribute.vi") -> (appended path=w507:path)
                n201 = Build Path(base path=w505, name or relative path="Write Expired.vi") -> (appended path=w502:path)
                n202 = Build Path(base path=w505, name or relative path="Write Error.vi") -> (appended path=w503:path)
                n203 = Build Array(w511, w510, w509, w508, w507, w501, w494, w502, w503) -> (w525:path[])
                n204 = for {
                  shift-right: [w550] -> w538
                  shift-left: w522 -> [w551]
                  tunnel: w520 -> [w549] mode=indexing
                  tunnel: w525 -> [w547] mode=indexing
                  n205 = invoke class="GObj" method="Replace"(reference=w549, error in=w551, "Path"=w547) -> (reference out=w548:refnum<vi>, error out=w550:errorcluster)  [unwired: 3 in, 4 out]
                  n206 = Close Reference(reference=w548) -> ()  [unwired: 1 in, 1 out]
                }
              }
              frame 6 {
                n207 = property class="LVClassLibrary"(reference=w572, error in=w573) -> (error out=w570:errorcluster, "Project"=w571:refnum<vi>)  [unwired: 1 out]
                n208 = property class="Project"(reference=w571, error in=w570) -> (reference out=w568:refnum<vi>, error out=w569:errorcluster, "Path"=w560:path)
                n209 = Strip Path(path=w560) -> (stripped path=w559:path)  [unwired: 1 out]
                n210 = Build Path(base path=w559, name or relative path="Packages") -> (appended path=w566:path)
                n211 = Close Reference(reference=w568) -> ()  [unwired: 1 in, 1 out]
                n212 = Build Path(base path=w566, name or relative path="CSPP_Core") -> (appended path=w552:path)
                n213 = Build Path(base path=w552, name or relative path="Messages") -> (appended path=w555:path)
                n214 = Build Path(base path=w555, name or relative path="CS++AcknowledgeMsg") -> (appended path=w554:path)
                n215 = Build Path(base path=w554, name or relative path="Read ReturnParameter.vi") -> (appended path=w553:path)
                n216 = for {
                  tunnel: w575 -> [w582]
                  tunnel: string[] ["Dummy Read ReturnParameter.vi"] -> [w576] mode=indexing
                  shift-right: [w578] -> w558
                  shift-left: w569 -> [w579]
                  tunnel: [w577] -> w556 mode=indexing
                  n217 = call <vilib>:"TRef Find Object By Label.vi"("Label"=w576, "Traverse Target"=TRef_TravTarget."BD", "error in (no error)"=w579, "Class Name"="SubVI", "VI Ref"=w582) -> ("error out"=w578:errorcluster, "Found Obj Ref"=w577:refnum<vi>)  [unwired: 3 in, 2 out]
                }
                n218 = Build Array(w553) -> (w561:path[])
                n219 = for {
                  shift-right: [w586] -> w574
                  shift-left: w558 -> [w587]
                  tunnel: w556 -> [w585] mode=indexing
                  tunnel: w561 -> [w583] mode=indexing
                  n220 = invoke class="GObj" method="Replace"(reference=w585, error in=w587, "Path"=w583) -> (reference out=w584:refnum<vi>, error out=w586:errorcluster)  [unwired: 3 in, 4 out]
                  n221 = Close Reference(reference=w584) -> ()  [unwired: 1 in, 1 out]
                }
              }
            }
          }
          frame "RedoWiring" {
            # "Case 9: For unknown reasons in the Asynch Case some wires have to be redone manually"
            n222 = case shown="4, 5" w591 {
              tunnel: [w593 w663] -> w590
              tunnel: w589 -> [w593 w693]
              tunnel: w588 -> [_ w694]
              frame Default {
              }
              frame 4, 5 {
                w603 = "Expired?"
                w661 = refnum<vi> refnum  # ControlTerminal
                n223 = for {
                  tunnel: w694 -> [w735]
                  tunnel: string[] ["Write AcknowledgeMsg.vi", "Error Cluster from Error Code.vi", "Write Error.vi", "Do.vi"] -> [w731] mode=indexing
                  shift-right: [w728] -> w673
                  shift-left: w693 -> [w732]
                  tunnel: [w726] -> w667 mode=indexing
                  w727 = refnum<vi> refnum  # SubVI
                  n224 = call <vilib>:"TRef Find Object By Label.vi"("Label"=w731, "Traverse Target"=TRef_TravTarget."BD", "error in (no error)"=w732, "Class Name"="SubVI", "VI Ref"=w735) -> ("error out"=w730:errorcluster, "Found Obj Ref"=w729:refnum<vi>)  [unwired: 3 in, 2 out]
                  n225 = To More Specific Class(target class=w727, reference=w729, error in=w730) -> (specific class reference=w726:refnum<vi>, error out=w728:errorcluster)
                }
                n226 = for {
                  tunnel: w694 -> [w725]
                  tunnel: string[] ["ErrorCode", "ErrorMsg"] -> [w721] mode=indexing
                  shift-right: [w719] -> w672
                  shift-left: w693 -> [w722]
                  tunnel: [w716] -> w654 mode=indexing
                  w720 = refnum<vi> refnum  # Constant
                  n227 = call <vilib>:"TRef Find Object By Label.vi"("Label"=w721, "Traverse Target"=TRef_TravTarget."BD", "error in (no error)"=w722, "Class Name"="Constant", "VI Ref"=w725) -> ("error out"=w718:errorcluster, "Found Obj Ref"=w717:refnum<vi>)  [unwired: 3 in, 2 out]
                  n228 = To More Specific Class(target class=w720, reference=w717, error in=w718) -> (specific class reference=w716:refnum<vi>, error out=w719:errorcluster)
                }
                n229 = for {
                  tunnel: w694 -> [w715]
                  tunnel: string[] ["Actor out", "error out"] -> [w712] mode=indexing
                  shift-right: [w711] -> w671
                  shift-left: w693 -> [w713]
                  tunnel: [w708] -> w660 mode=indexing
                  tunnel: w661 -> [w707]
                  tunnel: "ControlTerminal" -> [w706]
                  tunnel: [w705] -> w622
                  n230 = call <vilib>:"TRef Find Object By Label.vi"("Label"=w712, "Traverse Target"=TRef_TravTarget."BD", "error in (no error)"=w713, "Class Name"=w706, "VI Ref"=w715) -> ("error out"=w710:errorcluster, "Found Obj Ref"=w709:refnum<vi>, "dup VI Ref"=w705:refnum<vi>)  [unwired: 3 in, 1 out]
                  n231 = To More Specific Class(target class=w707, reference=w709, error in=w710) -> (specific class reference=w708:refnum<vi>, error out=w711:errorcluster)
                }
                n232 = Index Array(array=w654, index #1=0 ("index"), index #2=1 ("index")) -> (element #1=w653:refnum<vi>, element #2=w652:refnum<vi>)
                n233 = Merge Errors(w673, w672, w671) -> (w636:errorcluster)
                n234 = Index Array(array=w667, index #1=3 ("index"), index #2=1 ("index"), index #3=2 ("index"), index #4=0 ("index")) -> (element #1=w690:refnum<vi>, element #2=w679:refnum<vi>, element #3=w678:refnum<vi>, element #4=w635:refnum<vi>)
                n235 = Index Array(array=w660, index #1=0 ("index"), index #2=1 ("index")) -> (element #1=w688:refnum<vi>, element #2=w685:refnum<vi>)
                n236 = Build Array (concatenate)(w667, w654, w660) -> (w666:refnum<vi>[])
                n237 = property class="SubVI"(reference=w635, error in=w636) -> (error out=w634:errorcluster, "Terms[]"=w632:refnum<vi>[])  [unwired: 1 out]
                n238 = property class="SubVI"(reference=w690, error in=w636) -> (error out=w670:errorcluster, "Terms[]"=w665:refnum<vi>[])  [unwired: 1 out]
                n239 = property class="SubVI"(reference=w679, error in=w636) -> (error out=w669:errorcluster, "Terms[]"=w629:refnum<vi>[])  [unwired: 1 out]
                n240 = property class="SubVI"(reference=w678, error in=w636) -> (error out=w668:errorcluster, "Terms[]"=w664:refnum<vi>[])  [unwired: 1 out]
                n241 = property class="Const"(reference=w653, error in=w636) -> (error out=w648:errorcluster, "Terminal"=w642:refnum<vi>)  [unwired: 1 out]
                n242 = property class="Const"(reference=w652, error in=w636) -> (error out=w649:errorcluster, "Terminal"=w645:refnum<vi>)  [unwired: 1 out]
                n243 = property class="CtrlTerm"(reference=w688, error in=w636) -> (error out=w650:errorcluster, "Control"=w659:refnum<vi>)  [unwired: 1 out]
                n244 = property class="CtrlTerm"(reference=w685, error in=w636) -> (error out=w651:errorcluster, "Control"=w658:refnum<vi>)  [unwired: 1 out]
                n245 = Merge Errors(w634, w670, w669, w668, w648, w649, w650, w651) -> (w623:errorcluster)
                n246 = property class="Ctl"(reference=w659) -> (error out=w624:errorcluster, "Terminal"=w633:refnum<vi>)  [unwired: 1 in, 1 out]
                n247 = Index Array(array=w632, index #1=3 ("index"), index #2=10 ("index")) -> (element #1=w630:refnum<vi>, element #2=w620:refnum<vi>)
                n248 = Index Array(array=w665, index #1=2 ("index"), index #2=0 ("index"), index #3=11 ("index"), index #4=8 ("index"), index #5=10 ("index")) -> (element #1=w686:refnum<vi>, element #2=w683:refnum<vi>, element #3=w638:refnum<vi>, element #4=w627:refnum<vi>, element #5=w618:refnum<vi>)
                n249 = Index Array(array=w629, index=0) -> (element=w675:refnum<vi>)
                n250 = Index Array(array=w629, index=10) -> (element=w641:refnum<vi>)
                n251 = Index Array(array=w629, index=11) -> (element=w640:refnum<vi>)
                n252 = Index Array(array=w664, index=10) -> (element=w674:refnum<vi>)
                n253 = property class="Ctl"(reference=w658) -> (error out=w647:errorcluster, "Terminal"=w646:refnum<vi>)  [unwired: 1 in, 1 out]
                n254 = Build Array (concatenate)(w666, w665, w629, w664, w659, w658, w632, w633, w642, w645, w646) -> (w626:refnum<vi>[])
                n255 = call "GetCaseTerm.vi"("error in (no error)"=w623, "CaseStructureName"=w603, "WireLabel"="actor", "VI Ref"=w622) -> ("error out"=w604:errorcluster, "Open Refs"=w608:refnum<vi>[], "Terminal Ref"=w602:refnum<vi>)  [unwired: 4 in, 1 out]
                n256 = call "GetCaseTerm.vi"("error in (no error)"=w623, "CaseStructureName"=w603, "WireLabel"="msg", "VI Ref"=w622) -> ("error out"=w605:errorcluster, "Open Refs"=w607:refnum<vi>[], "Terminal Ref"=w601:refnum<vi>)  [unwired: 4 in, 1 out]
                n257 = call "GetCaseTerm.vi"("error in (no error)"=w623, "CaseStructureName"=w603, "WireLabel"="error", "VI Ref"=w622) -> ("error out"=w606:errorcluster, "Open Refs"=w609:refnum<vi>[], "Terminal Ref"=w610:refnum<vi>)  [unwired: 4 in, 1 out]
                n258 = Merge Errors(w623, w604, w605, w606, w624, w647) -> (w614:errorcluster)
                n259 = Build Array (concatenate)(w626, w608, w607, w609) -> (w625:refnum<vi>[])
                n260 = Build Array(w686, w633) -> (w617:refnum<vi>[])
                n261 = Build Array(w683, w646) -> (w616:refnum<vi>[])
                n262 = Build Array(w675, w674) -> (w615:refnum<vi>[])
                n263 = Build Array(w638, w630) -> (w611:refnum<vi>[])
                n264 = Build Array(w627, w610) -> (w600:refnum<vi>[])
                n265 = Build Array(w642, w640) -> (w613:refnum<vi>[])
                n266 = Build Array(w645, w641) -> (w612:refnum<vi>[])
                n267 = Build Array(w602, w618) -> (w599:refnum<vi>[])
                n268 = Build Array(w601, w620) -> (w598:refnum<vi>[])
                n269 = Build Array(w617, w616, w615, w613, w612, w611, w599, w598, w600) -> (w594:refnum<vi>[][])
                n270 = for {
                  shift-right: [w700] -> w662
                  shift-left: w614 -> [w701]
                  tunnel: w594 -> [w699] mode=indexing
                  n271 = Index Array(array=w699) -> (element #1=w698:refnum<vi>, element #2=w697:refnum<vi>)  [unwired: 2 in]
                  n272 = invoke class="Term" method="Connect Wire"(reference=w698, error in=w701, "Wire Source"=w697) -> (error out=w700:errorcluster)  [unwired: 4 in, 6 out]
                }
                n273 = flat-sequence {
                  tunnel: [w703] -> w663
                  tunnel: w662 -> [w703]
                  tunnel: w625 -> [w702]
                  frame #0 {
                    n274 = for {
                      tunnel: w702 -> [w704] mode=indexing
                      n275 = Close Reference(reference=w704) -> ()  [unwired: 1 in, 1 out]
                    }
                  }
                }
              }
            }
          }
          frame "Connect MethodOut to Bundler" {
            # "Case 10: In case of an Asynch Msg connect outputs of Action method to the bundler"
            n276 = case shown="4, 5" w740 {
              tunnel: [w744 w757] -> w742
              tunnel: w741 -> [w744 w757]
              tunnel: w739 -> [_ w752]
              tunnel: w738 -> [w743 w751]
              tunnel: w737 -> [_ w758]
              tunnel: [w743 w749] -> w736
              frame Default {
              }
              frame 4, 5 {
                w759 = refnum<vi> refnum  # Bundler
                n277 = Unbundle By Name(w758) -> ("Out-Terminals"=w753:T8)
                n278 = call <vilib>:"TRef Find Object By Label.vi"("Label"="Out-Bundler", "Traverse Target"=TRef_TravTarget."BD", "error in (no error)"=w751, "Class Name"="Bundler", "VI Ref"=w752) -> ("error out"=w761:errorcluster, "Found Obj Ref"=w760:refnum<vi>, "dup VI Ref"=w750:refnum<vi>)  [unwired: 3 in, 1 out]
                n279 = Array Size(array=w753) -> (size(s)=w746:i32)
                n280 = for {
                  tunnel: w753 -> [w849] mode=indexing
                  tunnel: [w848] -> w756 mode=indexing
                  n281 = Unbundle By Name(w849) -> ("Terminal"=w848:i32)
                }
                n282 = To More Specific Class(target class=w759, reference=w760, error in=w761) -> (specific class reference=w755:refnum<vi>, error out=w754:errorcluster)
                n283 = Equal To 0?(x=w746) -> (x = 0?=w745:bool)
                n284 = case "No output?" shown="True" w745 {
                  tunnel: w757 -> [w780 _]
                  tunnel: w756 -> [w779 _]
                  tunnel: w755 -> [w778 w810]
                  tunnel: w754 -> [w777 w828]
                  tunnel: w746 -> [w776 _]
                  tunnel: w750 -> [w770 w829]
                  tunnel: [w769 w811] -> w748
                  tunnel: [w765 w807] -> w747
                  frame False {
                    # "4,5"
                    n285 = property class="Bundler"(reference=w778, error in=w777, "InputCnt"=w776) -> (reference out=w775:refnum<vi>, error out=w774:errorcluster)
                    n286 = property class="Bundler"(reference=w775, error in=w774) -> (reference out=w772:refnum<vi>, error out=w773:errorcluster, "InputTerms[]"=w771:refnum<vi>[])
                    n287 = for {
                      tunnel: w780 -> [w805]
                      tunnel: w779 -> [w804] mode=indexing
                      tunnel: w771 -> [w802] mode=indexing
                      shift-right: [w783] -> w769
                      shift-left: w773 -> [w801]
                      tunnel: w770 -> [w794]
                      tunnel: [w782] -> w767 mode=concatenating
                      tunnel: [w781] -> w766 mode=indexing
                      i -> [w798]
                      w787 = refnum<vi> refnum  # ConditionalTunnel
                      n288 = Index Array(array=w805, index=w804) -> (element=w803:refnum<vi>)
                      n289 = Number To Decimal String(number=w798) -> (decimal integer string=w796:string)  [unwired: 1 in]
                      n290 = invoke class="Term" method="Connect Wire"(reference=w802, error in=w801, "Wire Source"=w803) -> (reference out=w800:refnum<vi>, error out=w799:errorcluster)  [unwired: 4 in, 5 out]
                      n291 = Concatenate Strings("L", w796) -> (w793:string)
                      n292 = property class="Term"(reference=w800, error in=w799, "Wire.Label.Text"=w793) -> (error out=w795:errorcluster)  [unwired: 1 out]
                      n293 = call "GetCaseTerm.vi"("error in (no error)"=w795, "CaseStructureName"="Error Case", "WireLabel"=w793, "VI Ref"=w794) -> ("error out"=w788:errorcluster, "Open Refs"=w782:refnum<vi>[], "Terminal Ref"=w789:refnum<vi>)  [unwired: 4 in, 1 out]
                      n294 = property class="OutrTerm"(reference=w789, error in=w788) -> (error out=w791:errorcluster, "Tunnel"=w790:refnum<vi>)  [unwired: 1 out]
                      n295 = To More Specific Class(target class=w787, reference=w790, error in=w791) -> (specific class reference=w785:refnum<vi>, error out=w786:errorcluster)
                      n296 = property class="CondTun"(reference=w785, error in=w786, "UseDefault"=TRUE ("Use Default if Unwired")) -> (reference out=w781:refnum<vi>, error out=w783:errorcluster)
                    }
                    n297 = Build Array (concatenate)(w772, w771) -> (w768:refnum<vi>[])
                    n298 = Build Array (concatenate)(w768, w767, w766) -> (w765:refnum<vi>[])
                  }
                  frame True {
                    w826 = refnum<vi> refnum  # SubVI
                    # "Delete Out-Bundle and Write VI and reconnect wire"
                    n299 = call <vilib>:"TRef Find Object By Label.vi"("Label"="Variant to Attribute.vi", "Traverse Target"=TRef_TravTarget."BD", "error in (no error)"=w828, "Class Name"="SubVI", "VI Ref"=w829) -> ("error out"=w827:errorcluster, "Found Obj Ref"=w830:refnum<vi>)  [unwired: 3 in, 2 out]
                    n300 = To More Specific Class(target class=w826, reference=w830, error in=w827) -> (specific class reference=w824:refnum<vi>, error out=w823:errorcluster)
                    n301 = property class="SubVI"(reference=w824, error in=w823) -> (reference out=w809:refnum<vi>, error out=w817:errorcluster, "Terms[]"=w806:refnum<vi>[])
                    n302 = Build Array(w810, w809) -> (w808:refnum<vi>[])
                    n303 = Index Array(array=w806, index #1=3 ("index"), index #2=11 ("index")) -> (element #1=w820:refnum<vi>, element #2=w819:refnum<vi>)
                    n304 = Build Array(w820, w819) -> (w818:refnum<vi>[])
                    n305 = for {
                      tunnel: w818 -> [w842] mode=indexing
                      shift-right: [w838] -> w813
                      shift-left: w817 -> [w841]
                      tunnel: [w839] -> w816 mode=indexing
                      n306 = property class="Term"(reference=w842, error in=w841) -> (error out=w838:errorcluster, "Wire.Terms[]"=w840:refnum<vi>[])  [unwired: 1 out]
                      n307 = Not Equal?(x=w840, y=w842) -> (x != y?=w837:bool[])
                      n308 = for {
                        tunnel: w837 -> [w844] mode=indexing
                        tunnel: [w843] -> w836
                        i -> [w843]
                        stop <- w844 stop-if-true
                      }
                      n309 = Index Array(array=w840, index=w836) -> (element=w839:refnum<vi>)
                    }
                    n310 = Index Array(array=w816) -> (element #1=w815:refnum<vi>, element #2=w814:refnum<vi>)  [unwired: 2 in]
                    n311 = invoke class="Term" method="Connect Wire"(reference=w815, error in=w813, "Wire Source"=w814) -> (error out=w812:errorcluster)  [unwired: 4 in, 6 out]
                    n312 = for {
                      shift-right: [w834] -> w811
                      shift-left: w812 -> [w835]
                      tunnel: w808 -> [w833] mode=indexing
                      n313 = invoke class="Node" method="Delete"(reference=w833, error in=w835) -> (error out=w834:errorcluster)  [unwired: 1 in, 2 out]
                    }
                    n314 = Build Array (concatenate)(w808, w806) -> (w807:refnum<vi>[])
                  }
                }
                n315 = flat-sequence {
                  tunnel: w747 -> [w846]
                  tunnel: [w845] -> w749
                  tunnel: w748 -> [w845]
                  frame #0 {
                    n316 = for {
                      tunnel: w846 -> [w847] mode=indexing
                      n317 = Close Reference(reference=w847) -> ()  [unwired: 1 in, 1 out]
                    }
                  }
                }
              }
            }
          }
          frame "Delete AsynchAndNoPara" {
            # "Case 11: In case of an Asynch Msg and no Caller parameters some functions have to be deleted."
            n318 = Unbundle By Name(w853) -> ("In-Terminals"=w852:T8)
            n319 = Array Size(array=w852) -> (size(s)=w851:i32)
            n320 = Equal To 0?(x=w851) -> (x = 0?=w850:bool)
            n321 = case shown="True" w850 {
              tunnel: w857 -> [_ w863]
              tunnel: [w859 w862] -> w856
              tunnel: w855 -> [w859 w861]
              tunnel: w854 -> [_ w860]
              frame False {
              }
              frame True {
                n322 = case shown="4, 5" w863 {
                  tunnel: [w864 w867] -> w862
                  tunnel: w861 -> [w864 w883]
                  tunnel: w860 -> [_ w885]
                  frame Default {
                  }
                  frame 4, 5 {
                    w897 = refnum<vi> refnum  # Function
                    w910 = refnum<vi> refnum  # SubVI
                    # "4,5"
                    n323 = call <vilib>:"TRef Find Object By Label.vi"("Label"="Type", "Traverse Target"=TRef_TravTarget."BD", "error in (no error)"=w883, "Class Name"="ClusterConstant", "VI Ref"=w885) -> ("error out"=w880:errorcluster, "Found Obj Ref"=w881:refnum<vi>, "dup VI Ref"=w884:refnum<vi>)  [unwired: 3 in, 1 out]
                    n324 = invoke class="GObj" method="Delete"(reference=w881, error in=w880) -> (reference out=w875:refnum<vi>, error out=w879:errorcluster)  [unwired: 1 in, 1 out]
                    n325 = call <vilib>:"TRef Find Object By Label.vi"("Label"="Read CallerParameter.vi", "Traverse Target"=TRef_TravTarget."BD", "error in (no error)"=w879, "Class Name"="SubVI", "VI Ref"=w884) -> ("error out"=w911:errorcluster, "Found Obj Ref"=w912:refnum<vi>)  [unwired: 3 in, 2 out]
                    n326 = call <vilib>:"TRef Find Object By Label.vi"("Label"="Variant To Data", "Traverse Target"=TRef_TravTarget."BD", "error in (no error)"=w879, "Class Name"="Function", "VI Ref"=w884) -> ("error out"=w896:errorcluster, "Found Obj Ref"=w895:refnum<vi>)  [unwired: 3 in, 2 out]
                    n327 = To More Specific Class(target class=w910, reference=w912, error in=w911) -> (specific class reference=w908:refnum<vi>, error out=w907:errorcluster)
                    n328 = To More Specific Class(target class=w897, reference=w895, error in=w896) -> (specific class reference=w899:refnum<vi>, error out=w900:errorcluster)
                    n329 = property class="SubVI"(reference=w908, error in=w907) -> (reference out=w874:refnum<vi>, error out=w878:errorcluster, "Terms[]"=w871:refnum<vi>[])
                    n330 = property class="Func"(reference=w899, error in=w900) -> (reference out=w872:refnum<vi>, error out=w876:errorcluster, "Terms[]"=w870:refnum<vi>[])
                    n331 = Index Array(array=w871, index #1=3 ("index"), index #2=11 ("index")) -> (element #1=w904:refnum<vi>, element #2=w903:refnum<vi>)
                    n332 = Index Array(array=w870, index #1=0 ("index"), index #2=1 ("index")) -> (element #1=w891:refnum<vi>, element #2=w892:refnum<vi>)
                    n333 = Build Array(w904, w903) -> (w902:refnum<vi>[])
                    n334 = Build Array(w891, w892) -> (w888:refnum<vi>[])
                    n335 = Build Array(w874, w872) -> (w873:refnum<vi>[])
                    n336 = Merge Errors(w878, w876) -> (w877:errorcluster)
                    n337 = Build Array(w902, w888) -> (w901:refnum<vi>[][])
                    n338 = for {
                      tunnel: w901 -> [w922] mode=indexing
                      tunnel: w873 -> [w921] mode=indexing
                      shift-right: [w919] -> w866
                      shift-left: w877 -> [w923]
                      tunnel: [w918] -> w868 mode=indexing
                      tunnel: [w917] -> w869 mode=concatenating
                      n339 = for {
                        tunnel: w922 -> [w934] mode=indexing
                        shift-right: [w931] -> w926
                        shift-left: w923 -> [w933]
                        tunnel: [w932] -> w927 mode=indexing
                        tunnel: [w928] -> w917 mode=concatenating
                        n340 = property class="Term"(reference=w934, error in=w933) -> (error out=w931:errorcluster, "Wire.Terms[]"=w928:refnum<vi>[])  [unwired: 1 out]
                        n341 = Not Equal?(x=w928, y=w934) -> (x != y?=w930:bool[])
                        n342 = for {
                          tunnel: w930 -> [w936] mode=indexing
                          tunnel: [w935] -> w929
                          i -> [w935]
                          stop <- w936 stop-if-true
                        }
                        n343 = Index Array(array=w928, index=w929) -> (element=w932:refnum<vi>)
                      }
                      n344 = Index Array(array=w927) -> (element #1=w925:refnum<vi>, element #2=w924:refnum<vi>)  [unwired: 2 in]
                      n345 = invoke class="Term" method="Connect Wire"(reference=w925, error in=w926, "Wire Source"=w924) -> (error out=w920:errorcluster)  [unwired: 4 in, 6 out]
                      n346 = invoke class="Node" method="Delete"(reference=w921, error in=w920) -> (reference out=w918:refnum<vi>, error out=w919:errorcluster)  [unwired: 1 in, 1 out]
                    }
                    n347 = Build Array (concatenate)(w875, w871, w870, w869, w868) -> (w865:refnum<vi>[])
                    n348 = flat-sequence {
                      tunnel: [w916] -> w867
                      tunnel: w866 -> [w916]
                      tunnel: w865 -> [w915]
                      frame #0 {
                        n349 = Close Reference(reference=w915) -> ()  [unwired: 1 in, 1 out]
                      }
                    }
                  }
                }
              }
            }
          }
          frame "DeleteBoolDIMConversion" {
            # "Case 12: In the case of DIM a boolean will arrive as an I16. This is already included in the two PV Do.vis. But it has to be removed if the data is not simple boolean."
            n350 = case shown="2, 3" w940 {
              tunnel: [w943 w949] -> w939
              tunnel: w938 -> [w943 w970]
              tunnel: w937 -> [_ w971]
              frame Default {
              }
              frame 2, 3 {
                w965 = refnum<vi> refnum  # Unbundler
                n351 = call <vilib>:"TRef Find Object By Label.vi"("Label"="Pre-Unbundler" ("Class Name"), "Traverse Target"=TRef_TravTarget."BD", "error in (no error)"=w970, "Class Name"="Unbundler", "VI Ref"=w971) -> ("error out"=w967:errorcluster, "Found Obj Ref"=w966:refnum<vi>, "dup VI Ref"=w952:refnum<vi>)  [unwired: 3 in, 1 out]
                n352 = To More Specific Class(target class=w965, reference=w966, error in=w967) -> (specific class reference=w963:refnum<vi>, error out=w964:errorcluster)
                n353 = property class="Unbundler"(reference=w963, error in=w964) -> (reference out=w953:refnum<vi>, error out=w960:errorcluster, "OutputTerms[]"=w962:refnum<vi>[])
                n354 = Close Reference(reference=w953) -> ()  [unwired: 1 in, 1 out]
                n355 = Index Array(array=w962) -> (element=w961:refnum<vi>)  [unwired: 1 in]
                n356 = Array Size(array=w962) -> (size(s)=w955:i32)
                n357 = Equal?(x=w955, y=1) -> (x = y?=w946:bool)
                n358 = property class="Term"(reference=w961, error in=w960) -> (error out=w958:errorcluster, "Data Type"=w959:variant)  [unwired: 1 out]
                n359 = call <vilib>:"Get Type Information.vi"("error in (no error)"=w958, "Variant"=w959) -> ("error out"=w951:errorcluster, "Type"=w957:T7)  [unwired: 5 in, 3 out]
                n360 = Equal?(x=Data_Type."Boolean" ("Type"), y=w957) -> (x = y?=w945:bool)
                n361 = stacked-sequence {
                  seq-local: [w972 _ _] -> [_ w1032 _]
                  seq-local: [_ w1028 _] -> [_ _ w1088]
                  tunnel: w952 -> [w977 w1031 w1086]
                  tunnel: w951 -> [w976 _ _]
                  tunnel: "Function" ("Class Name") -> [w975 w1030 _]
                  tunnel: [_ _ w1087] -> w949
                  tunnel: "Constant" ("Class Name") -> [w974 w1029 _]
                  tunnel: w946 -> [w973 w1034 w1089]
                  tunnel: w945 -> [_ w1035 _]
                  tunnel: "ClusterConstant" ("Class Name") -> [_ _ w1085]
                  frame #0 {
                    n362 = case shown="True" w973 {
                      tunnel: w977 -> [_ w996]
                      tunnel: w976 -> [w978 w994]
                      tunnel: w975 -> [_ _]
                      tunnel: [w978 w999] -> w972
                      tunnel: w974 -> [_ _]
                      frame False {
                        # "Cluster needed ==> Do nothing"
                      }
                      frame True {
                        w993 = refnum<vi> refnum  # Unbundler
                        w1011 = refnum<vi> refnum  # Bundler
                        w1008 = refnum<vi> refnum  # Unbundler
                        w995 = TRef_TravTarget."BD" ("Traverse Target")
                        # "Only one parameter => Delete Pre-Bundler etc."
                        n363 = call <vilib>:"TRef Find Object By Label.vi"("Label"="Main-Unbundler" ("Class Name"), "Traverse Target"=w995, "error in (no error)"=w994, "Class Name"="Unbundler", "VI Ref"=w996) -> ("error out"=w992:errorcluster, "Found Obj Ref"=w991:refnum<vi>)  [unwired: 3 in, 2 out]
                        n364 = call <vilib>:"TRef Find Object By Label.vi"("Label"="Pre-Bundler" ("Class Name"), "Traverse Target"=w995, "error in (no error)"=w994, "Class Name"="Bundler", "VI Ref"=w996) -> ("error out"=w1015:errorcluster, "Found Obj Ref"=w1014:refnum<vi>)  [unwired: 3 in, 2 out]
                        n365 = call <vilib>:"TRef Find Object By Label.vi"("Label"="Pre-Unbundler" ("Class Name"), "Traverse Target"=w995, "error in (no error)"=w994, "Class Name"="Unbundler", "VI Ref"=w996) -> ("error out"=w1009:errorcluster, "Found Obj Ref"=w1010:refnum<vi>)  [unwired: 3 in, 2 out]
                        n366 = To More Specific Class(target class=w1011, reference=w1014, error in=w1015) -> (specific class reference=w1012:refnum<vi>, error out=w1013:errorcluster)
                        n367 = To More Specific Class(target class=w993, reference=w991, error in=w992) -> (specific class reference=w990:refnum<vi>, error out=w989:errorcluster)
                        n368 = To More Specific Class(target class=w1008, reference=w1010, error in=w1009) -> (specific class reference=w1007:refnum<vi>, error out=w1006:errorcluster)
                        n369 = property class="Unbundler"(reference=w990, error in=w989) -> (reference out=w984:refnum<vi>, error out=w985:errorcluster, "Terms[]"=w982:refnum<vi>[])
                        n370 = property class="Unbundler"(reference=w990, error in=w989) -> (error out=w979:errorcluster, "OutputTerms[]"=w981:refnum<vi>[])  [unwired: 1 out]
                        n371 = property class="Bundler"(reference=w1012, error in=w1013) -> (reference out=w1016:refnum<vi>, error out=w1020:errorcluster, "Terms[]"=w1023:refnum<vi>[])
                        n372 = property class="Unbundler"(reference=w1007, error in=w1006) -> (reference out=w1025:refnum<vi>, error out=w1021:errorcluster, "OutputTerms[]"=w1024:refnum<vi>[])
                        n373 = Index Array(array=w982) -> (element=w988:refnum<vi>)  [unwired: 1 in]
                        n374 = Index Array(array=w981) -> (element=w987:refnum<vi>)  [unwired: 1 in]
                        n375 = Index Array(array=w1023) -> (element=w1017:refnum<vi>)  [unwired: 1 in]
                        n376 = Index Array(array=w1024) -> (element=w1018:refnum<vi>)  [unwired: 1 in]
                        n377 = Merge Errors(w1020, w1021) -> (w1019:errorcluster)
                        n378 = invoke class="Term" method="Connect Wire"(reference=w988, error in=w985, "Wire Source"=w987) -> (error out=w986:errorcluster)  [unwired: 4 in, 6 out]
                        n379 = invoke class="Term" method="Connect Wire"(reference=w1017, error in=w1019, "Wire Source"=w1018) -> (error out=w1022:errorcluster)  [unwired: 4 in, 6 out]
                        n380 = invoke class="Unbundler" method="Delete"(reference=w984, error in=w986) -> (reference out=w983:refnum<vi>, error out=w980:errorcluster)  [unwired: 1 in, 1 out]
                        n381 = invoke class="Bundler" method="Delete"(reference=w1016, error in=w1022) -> (reference out=w1026:refnum<vi>, error out=w1001:errorcluster)  [unwired: 1 in, 1 out]
                        n382 = Build Array (concatenate)(w983, w982, w981, w1023, w1024, w1025, w1026) -> (w1000:refnum<vi>[])
                        n383 = Merge Errors(w980, w979, w1001) -> (w999:errorcluster)
                        n384 = for {
                          tunnel: w1000 -> [w1027] mode=indexing
                          tunnel: w999 -> [_]
                          n385 = Close Reference(reference=w1027) -> ()  [unwired: 1 in, 1 out]
                        }
                      }
                    }
                  }
                  frame #1 {
                    n386 = And(x=w1035, y=w1034) -> (x .and. y?=w1033:bool)
                    n387 = case shown="False" w1033 {
                      tunnel: w1032 -> [w1037 w1084]
                      tunnel: [w1040 w1084] -> w1028
                      tunnel: w1031 -> [w1039 _]
                      tunnel: w1030 -> [w1038 _]
                      tunnel: w1029 -> [w1036 _]
                      frame False {
                        w1041 = TRef_TravTarget."BD" ("Traverse Target")
                        w1066 = refnum<vi> refnum  # Function
                        w1072 = refnum<vi> refnum  # Function
                        # "It is not only one boolean ==> Delete 2nd TypeCast"
                        n388 = call <vilib>:"TRef Find Object By Label.vi"("Label"="I16-Conversion" ("Class Name"), "Traverse Target"=w1041, "error in (no error)"=w1037, "Class Name"=w1038, "VI Ref"=w1039) -> ("error out"=w1080:errorcluster, "Found Obj Ref"=w1081:refnum<vi>)  [unwired: 3 in, 2 out]
                        n389 = call <vilib>:"TRef Find Object By Label.vi"("Label"="I16-Conversion-Constant" ("Class Name"), "Traverse Target"=w1041, "error in (no error)"=w1037, "Class Name"=w1036, "VI Ref"=w1039) -> ("error out"=w1079:errorcluster, "Found Obj Ref"=w1078:refnum<vi>)  [unwired: 3 in, 2 out]
                        n390 = call <vilib>:"TRef Find Object By Label.vi"("Label"="I16-Comp0" ("Class Name"), "Traverse Target"=w1041, "error in (no error)"=w1037, "Class Name"=w1038, "VI Ref"=w1039) -> ("error out"=w1074:errorcluster, "Found Obj Ref"=w1075:refnum<vi>)  [unwired: 3 in, 2 out]
                        n391 = call <vilib>:"TRef Find Object By Label.vi"("Label"="I16-Select" ("Class Name"), "Traverse Target"=w1041, "error in (no error)"=w1037, "Class Name"=w1038, "VI Ref"=w1039) -> ("error out"=w1070:errorcluster, "Found Obj Ref"=w1071:refnum<vi>)  [unwired: 3 in, 2 out]
                        n392 = invoke class="GObj" method="Delete"(reference=w1081, error in=w1080) -> (reference out=w1045:refnum<vi>, error out=w1056:errorcluster)  [unwired: 1 in, 1 out]
                        n393 = invoke class="GObj" method="Delete"(reference=w1078, error in=w1079) -> (reference out=w1044:refnum<vi>, error out=w1054:errorcluster)  [unwired: 1 in, 1 out]
                        n394 = invoke class="GObj" method="Delete"(reference=w1075, error in=w1074) -> (reference out=w1043:refnum<vi>, error out=w1053:errorcluster)  [unwired: 1 in, 1 out]
                        n395 = To More Specific Class(target class=w1072, reference=w1071, error in=w1070) -> (specific class reference=w1069:refnum<vi>, error out=w1058:errorcluster)
                        n396 = property class="Func"(reference=w1069, error in=w1058) -> (reference out=w1050:refnum<vi>, error out=w1052:errorcluster, "Terms[]"=w1042:refnum<vi>[])
                        n397 = call <vilib>:"TRef Find Object By Label.vi"("Label"="MainSelect" ("Class Name"), "Traverse Target"=w1041, "error in (no error)"=w1037, "Class Name"=w1038, "VI Ref"=w1039) -> ("error out"=w1065:errorcluster, "Found Obj Ref"=w1064:refnum<vi>)  [unwired: 3 in, 2 out]
                        n398 = To More Specific Class(target class=w1066, reference=w1064, error in=w1065) -> (specific class reference=w1063:refnum<vi>, error out=w1062:errorcluster)
                        n399 = Index Array(array=w1042, index=3) -> (element=w1059:refnum<vi>)
                        n400 = property class="Func"(reference=w1063, error in=w1062) -> (reference out=w1046:refnum<vi>, error out=w1057:errorcluster, "Terms[]"=w1047:refnum<vi>[])
                        n401 = Index Array(array=w1047, index=1) -> (element=w1060:refnum<vi>)
                        n402 = Merge Errors(w1057, w1056, w1054, w1053, w1052) -> (w1055:errorcluster)
                        n403 = invoke class="Term" method="Connect Wire"(reference=w1060, error in=w1055, "Wire Source"=w1059) -> (error out=w1051:errorcluster)  [unwired: 4 in, 6 out]
                        n404 = invoke class="Func" method="Delete"(reference=w1050, error in=w1051) -> (reference out=w1049:refnum<vi>, error out=w1040:errorcluster)  [unwired: 1 in, 1 out]
                        n405 = Build Array (concatenate)(w1049, w1047, w1046, w1045, w1044, w1043, w1042) -> (w1048:refnum<vi>[])
                        n406 = for {
                          tunnel: w1040 -> [_]
                          tunnel: w1048 -> [w1083] mode=indexing
                          n407 = Close Reference(reference=w1083) -> ()  [unwired: 1 in, 1 out]
                        }
                      }
                      frame True {
                        # "It is only one boolean ==> 2nd Type Conversion needed"
                      }
                    }
                  }
                  frame #2 {
                    n408 = case shown="False" w1089 {
                      tunnel: w1088 -> [w1090 w1112]
                      tunnel: [w1090 w1098] -> w1087
                      tunnel: w1086 -> [_ w1113]
                      tunnel: w1085 -> [_ w1103]
                      frame False {
                        # "More parameters ==> Do nothing"
                      }
                      frame True {
                        w1116 = refnum<vi> refnum  # ClusterConstant
                        # "Only one paramater ==> Get TypeDescriptor out of Cluster"
                        n409 = call <vilib>:"TRef Find Object By Label.vi"("Label"="Type", "Traverse Target"=TRef_TravTarget."BD", "error in (no error)"=w1112, "Class Name"=w1103, "VI Ref"=w1113) -> ("error out"=w1115:errorcluster, "Found Obj Ref"=w1114:refnum<vi>, "dup VI Ref"=w1108:refnum<vi>)  [unwired: 3 in, 1 out]
                        n410 = property class="VI"(reference=w1108) -> ("Diagram"=w1107:refnum<vi>)  [unwired: 1 in, 2 out]
                        n411 = To More Specific Class(target class=w1116, reference=w1114, error in=w1115) -> (specific class reference=w1111:refnum<vi>, error out=w1110:errorcluster)
                        n412 = property class="ClustCnst"(reference=w1111, error in=w1110) -> (reference out=w1106:refnum<vi>, error out=w1104:errorcluster, "Elements[]"=w1094:refnum<vi>[])
                        n413 = Index Array(array=w1094) -> (element=w1109:refnum<vi>)  [unwired: 1 in]
                        n414 = invoke class="Const" method="Move"(reference=w1109, error in=w1104, "position"=T6 {"Left"=0, "Top"=0}, "owner"=w1107) -> (reference out=w1092:refnum<vi>, error out=w1105:errorcluster)  [unwired: 2 in, 4 out]
                        n415 = property class="ClustCnst"(reference=w1106, error in=w1105) -> (reference out=w1100:refnum<vi>, error out=w1101:errorcluster, "Terminal.Wire.Terms[]"=w1095:refnum<vi>[])
                        n416 = property class="Const"(reference=w1092) -> ("Terminal"=w1091:refnum<vi>)  [unwired: 1 in, 2 out]
                        n417 = Index Array(array=w1095) -> (element=w1102:refnum<vi>)  [unwired: 1 in]
                        n418 = invoke class="Term" method="Connect Wire"(reference=w1102, error in=w1101, "Wire Source"=w1091) -> (error out=w1099:errorcluster)  [unwired: 4 in, 6 out]
                        n419 = invoke class="ClustCnst" method="Delete"(reference=w1100, error in=w1099) -> (reference out=w1096:refnum<vi>, error out=w1098:errorcluster)  [unwired: 1 in, 1 out]
                        n420 = Build Array (concatenate)(w1096, w1095, w1094) -> (w1097:refnum<vi>[])
                        n421 = for {
                          tunnel: w1097 -> [w1119] mode=indexing
                          tunnel: w1098 -> [_]
                          n422 = Close Reference(reference=w1119) -> ()  [unwired: 1 in, 1 out]
                        }
                      }
                    }
                  }
                }
              }
            }
          }
        }
      }
      n423 = for {
        tunnel: w26 -> [w32] mode=indexing
        n424 = Close Reference(reference=w32) -> ()  [unwired: 1 in, 1 out]
      }
      n425 = invoke class="VI" method="BD.CleanUp"(reference=w25, error in=w28) -> (reference out=w13:refnum<vi>, error out=w11:errorcluster)  [unwired: 1 in, 1 out]
      n426 = invoke class="VI" method="Save.Instrument"(reference=w13, error in=w11) -> (reference out=w12:refnum<vi>, error out=w10:errorcluster)  [unwired: 4 in, 4 out]
      n427 = Close Reference(reference=w12, error in (no error)=w10) -> ()  [unwired: 1 out]
    }
    frame Error {
    }
  }
  "error out" <- w5
  "CS++Actor out" <- w3
